vi "MegaAwesome_9_21_12a_JW.vi"() -> ()   [LabVIEW 2011]
uses:
  MegaAwesome_States.ctl
  <vilib>/Utility/inputDevices.llb/keyboardAcquire.vi
  <vilib>/Utility/file.llb/Read From Spreadsheet File (string).vi
  <vilib>/Utility/file.llb/Write To Spreadsheet File (string).vi
panel:
  out "ROI Descriptor out":T1 {"Contours"."Type" items=["No Selection", "Point", "Line", "Rectangle", "Oval", "Polygon", "Freehand Region", "Annulus", "Unused2", "Unused3", "Broken Line", "Freehand Line", "Rotated Rectangle"]}
  out "ROI Descriptor":T1 {"Contours"."Type" items=["No Selection", "Point", "Line", "Rectangle", "Oval", "Polygon", "Freehand Region", "Annulus", "Unused2", "Unused3", "Broken Line", "Freehand Line", "Rotated Rectangle"]}
  in  "Slider Min":dbl=5.0
  in  "Slider Max":dbl=5.0
  out "Opj X Axis":string
  out "X Axis Display Type":string
  in  "Index-Sat":dbl=5.0
  in  "Index-Lin":dbl=5.0
  in  "IndexLog-Lin":dbl=5.0
  in  "IndexLog-Sat":dbl=5.0 caption="Num Pts"
  out "Lin Id-Log Used":dbl[](array[numeric])
  out "Lin-Vg Array-Log Used":dbl[](array[numeric])
  in  "New: Comments":string
  out "Save Array":string[][](array[string])
  out "Folder Index":i32 caption="Length"
  out "Sat Id-Used":dbl[](array[numeric])
  out "Sat Vg Array-Used":dbl[](array[numeric])
  out "Vg Array-Log-Used":dbl[](array[numeric])
  out "Sat Id-Log-Used":dbl[](array[numeric])
  out "Lin Id-Used":dbl[](array[numeric])
  out "Lin-Vg Array-Used":dbl[](array[numeric])
  out "Lin Vd":dbl
  out "Recorded Prop":T2
  out "Current State":T3
  in  "Main Tab Control":T4(tab)
  in  "Image Analysis?":bool
  in  "Image Folder":path
  out "Image File":path=path "D:/UserData/Desktop/Jeremy/WFU/Research/Programs/VI mods/Image Not Found.png"
  in  "Transfer File":path
  out "Transfer Folder":path
  out "Fabrication Prop":T5
  in  "Transport ?":bool
  out "Distances":dbl[](array[numeric])
  in  "Zoom":i16(slide)=-3 scale=-5.0..5.0
  in  "Magnification":u16(ring) items=["5x", "10x", "20x", "50x", "80x"]
  in  "Undo Button":bool
  in  "Remove Button":bool
  in  "Transfer Plots":T6(tab)=enum."Saturation"
  in  "Lin-Trans Slider":dbl(slide) step=1.0 scale=-40.0..40.0 scale format="%#_1p"
  out "Sqrt-Lin":cluster{dbl[], dbl[]}[](graph)
  in  "Sat-Trans Slider":dbl(slide) step=1.0 scale=-40.0..40.0 scale format="%#_1p"
  out "Sqrt-Sat":cluster{dbl[], dbl[]}[](graph)
  out "Raw- Lin":cluster{dbl[], dbl[]}[](graph)
  out "Raw- Sat":cluster{dbl[], dbl[]}[](graph)
  in  "Log Plots":enum32{"Linear", "Saturation", "Transport"}(tab)=enum."Saturation"
  in  "Lin-Log Slider":dbl(slide) step=1.0 scale=-40.0..40.0 scale format="%#_1p"
  out "Log-Lin":cluster{dbl[], dbl[]}[](graph)
  in  "Sat-Log Slider":dbl(slide) step=1.0 scale=-40.0..40.0 scale format="%#_1p"
  out "Sat-Log":cluster{dbl[], dbl[]}[](graph)
  out "Transport":cluster{dbl[], dbl[]}[](graph)
  in  "Manual Controls":T7
  in  "File Controls":T8
  out "Date Recorded":string="Date Recorded" caption="Measured"
  out "Data Name:":string
  out "Image Name":string
  out "Index":string
  out "Date Created":string caption="Fabricated"
  in  "Comments:":string
  out "Rec: Length":dbl caption="Length" format="%#_3g"
  out "Rec: Width":dbl caption="Width" format="%#_4g"
  out "Rec: Dielectric (d)":dbl caption="Dielectric (d)" format="%#_3g"
  in  "New: Dielectric":dbl
  in  "New: Length":dbl
  in  "New: Width":dbl
  out "Rec: Temp":dbl caption="Sample Temp" format="%.1f"
  in  "New: Temp":dbl format="%.1f"
  out "Image Out":T9(plugin-control)
  in  "Num Pts":dbl=5.0
  in  "Num Pts Log":dbl=5.0 caption="Num Pts"
  out "Recorded Values Cluster":T10
  out "Calculated Values Cluster":T10 caption="Recorded Values Cluster"
  out "Re-Calculated Values Cluster":T10 caption="Recorded Values Cluster"
  in  "Independant Variable:":string(combo)="Length (um):"
  out "Image Preview":T9(plugin-control)
  out "Total Width":dbl
  in  "No Image File":path=path "\\\\acad1\\physics/Jurchescu-group/JW-PD/Mega Awesome/Image Not Found.png"
  in  "Room Temp":dbl=294.0
  in  "Origin Project File":path=path "\\\\acad1\\physics/Jurchescu-group/JW-PD/Group Library/Origin Project Files/DeviceData_8_10_12a_JW.opj"
  in  "Transport Style Controls":T11={"Transport Line Size"=1, "Transport Line Color"=16772608} {"Transport Line Size" items=["Extra Small", "Small", "Medium", "Large", "Extra Large"]}
  # "Image Location"
  # "Recorded"
  # "Calculated"
  # "Re-Calculated"
  # "Manual"
  # "Used points display at y=0\nValues are wrong w/ slider"
  # "Slider\nDoesn't\nWork"
  # "Slider\nDoesn't\nWork"
  # "No new points displayed"
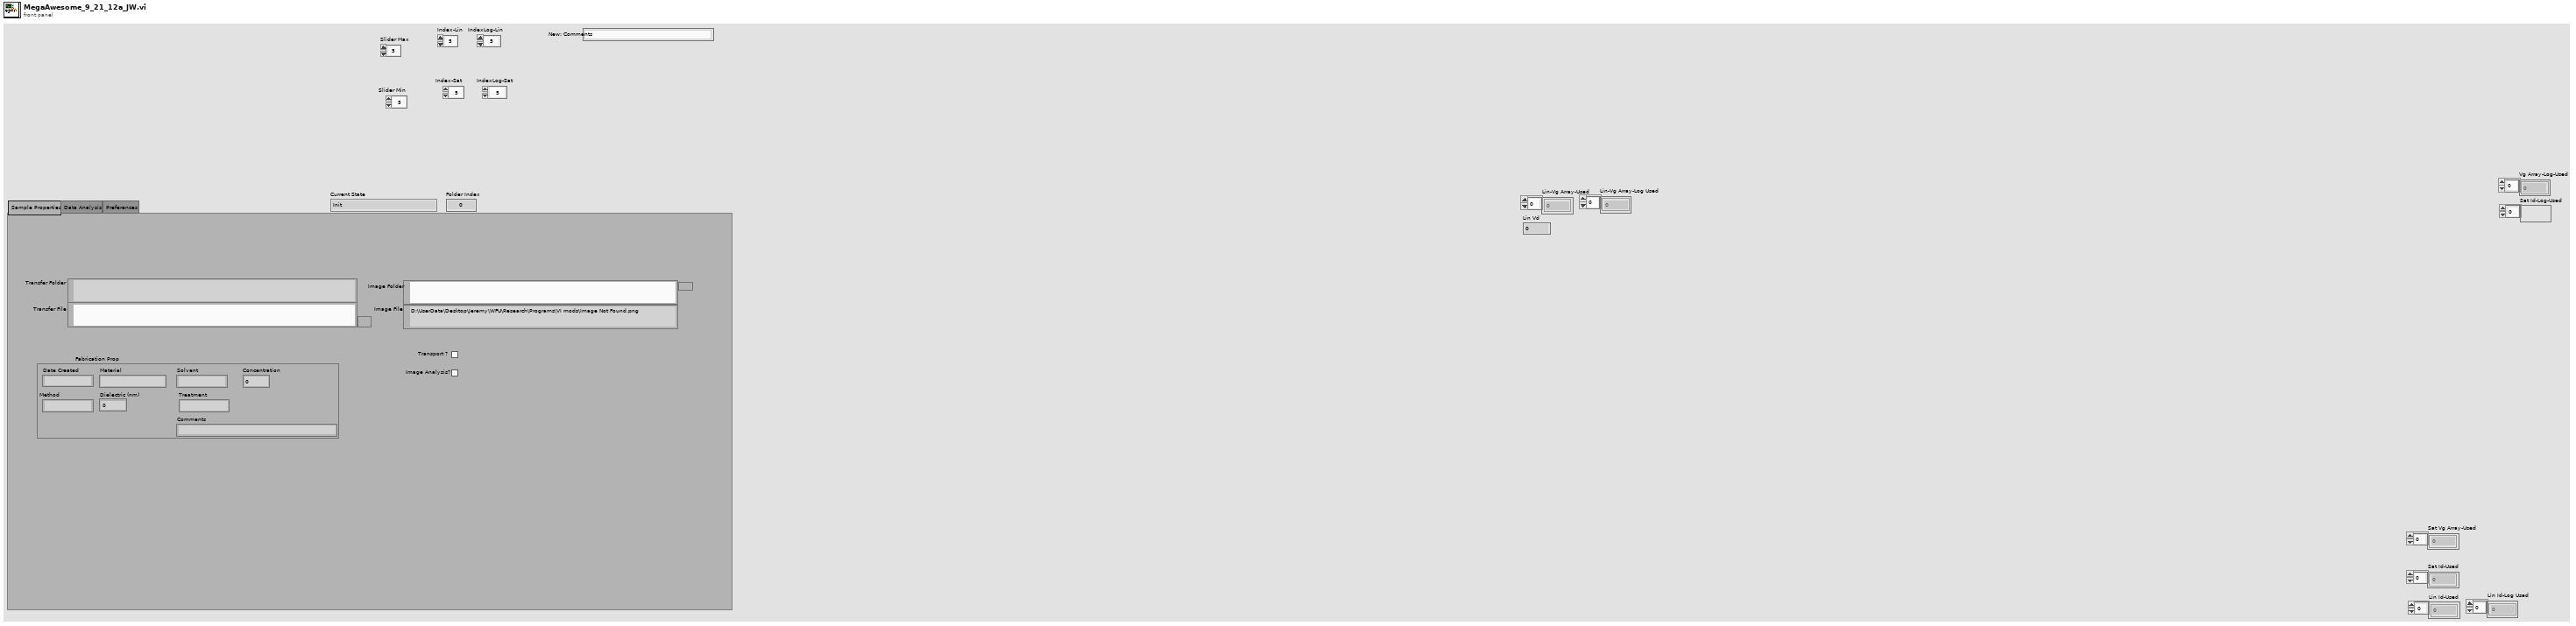
[diagram p1: front panel]
types:
  T1 = typedef "ROI Descriptor" = cluster{"Global Rectangle":i32[], "Contours":cluster{"ID":enum32{"External", "Internal"}, "Type":u32, "Coordinates":i32[]}[]}
  T2 = cluster{"Date Recorded":string, "Index":string, "Length":dbl, "Width":dbl, "Sample Temp":dbl}
  T3 = typedef "MegaAwesome_States.ctl" = enum16{"Init", "File Missing", "No Event", "Read Data", "Calculated Values", "Re-Calculated Values", "Next File", "Previous File", "Discard File", "Save", "Save Lines", "Export", "Exit"}
  T4 = enum32{"Sample Properties", "Data Analysis", "Preferences"}
  T5 = cluster{"Date Created":string, "Material":string, "Solvent":string, "Concentration":dbl, "Method":string, "Dielectric (nm)":dbl, "Treatment":string, "Comments":string}
  T6 = enum32{"Linear", "Saturation", "Raw-Linear", "Raw-Saturation"}
  T7 = cluster{"Manual-Temp":bool, "Manual-Width":bool, "Manuel-Length":bool, "Manuel-Dielectric":bool, "Manual Comments":bool}
  T8 = cluster{"Previous File":bool, "Discard ":bool, "Save Lines":bool, "Close":bool, "Next File ":bool, "Save":bool, "Save Next":bool, "Export":bool}
  T9 = typedef "IMAQ Image.ctl" = refnum<image>
  T10 = cluster{"Mobility-Sat":dbl, "Moblitity-Lin":dbl, "On/Off":dbl, "Off Current":dbl, "Vt-Sat":dbl, "STS":dbl, "Trap Density-VT":dbl, "Trap Density-STS":dbl}
  T11 = cluster{"Transport Line Size":u16, "Transport Line Color":u32}
  T12 = typedef "LVBoundsTypeDef.ctl" = cluster{"Width":u32, "Height":u32}
  T13 = cluster{"Global Rectangle":i32[], "Contours":cluster{"Contour Type":u32, "ROI Type":u32, "Points":i32[]}[]}
  T14 = cluster{"Contour Type":u32, "ROI Type":u32, "Points":i32[]}[]
  T15 = cluster{i32[], cluster{"Contour Type":u32, "ROI Type":u32, "Points":i32[]}[]}
  T16 = enum16{"0", "1", "2", "3", "4", "5", "6", "7", "8", "9", "A", "B", "C", "D", "E", "F", "G", "H", "I", "J", "K", "L", "M", "N", "O", "P", "Q", "R", "S", "T", "U", "V", "W", "X", "Y", "Z", "F1", "F2", "F3", "F4", "F5", "F6", "F7", "F8", "F9", "F10", "F11", "F12", "F13", "F14", "F15", "ADD", "BACK", "BACKSLASH", "CAPITAL", "COMMA", "DECIMAL", "DELETE", "DIVIDE", "DOWN", "END", "EQUALS", "ESCAPE", "GRAVE (`)", "HOME", "INSERT", "LBRACKET", "LCONTROL", "LEFT", "L ALT", "LSHIFT", "LWIN", "MINUS", "MULTIPLY", "NEXT", "NUMLOCK", "NUMPAD_0", "NUMPAD_1", "NUMPAD_2", "NUMPAD_3", "NUMPAD_4", "NUMPAD_5", "NUMPAD_6", "NUMPAD_7", "NUMPAD_8", "NUMPAD_9", "PAUSE", "PERIOD", "PRIOR (PG UP)", "RBRACKET", "RCONTROL", "RETURN", "RIGHT", "R ALT", "RSHIFT", "RWIN", "SCROLL", "SEMICOLON", "SLASH", "SPACE", "SUBTRACT", "TAB", "UP", "ENTER (num pad)", "' (quote)"}[]
  T17 = enum16{"0", "1", "2", "3", "4", "5", "6", "7", "8", "9", "A", "B", "C", "D", "E", "F", "G", "H", "I", "J", "K", "L", "M", "N", "O", "P", "Q", "R", "S", "T", "U", "V", "W", "X", "Y", "Z", "F1", "F2", "F3", "F4", "F5", "F6", "F7", "F8", "F9", "F10", "F11", "F12", "F13", "F14", "F15", "ADD", "BACK", "BACKSLASH", "CAPITAL", "COMMA", "DECIMAL", "DELETE", "DIVIDE", "DOWN", "END", "EQUALS", "ESCAPE", "GRAVE (`)", "HOME", "INSERT", "LBRACKET", "LCONTROL", "LEFT", "L ALT", "LSHIFT", "LWIN", "MINUS", "MULTIPLY", "NEXT", "NUMLOCK", "NUMPAD_0", "NUMPAD_1", "NUMPAD_2", "NUMPAD_3", "NUMPAD_4", "NUMPAD_5", "NUMPAD_6", "NUMPAD_7", "NUMPAD_8", "NUMPAD_9", "PAUSE", "PERIOD", "PRIOR (PG UP)", "RBRACKET", "RCONTROL", "RETURN", "RIGHT", "R ALT", "RSHIFT", "RWIN", "SCROLL", "SEMICOLON", "SLASH", "SPACE", "SUBTRACT", "TAB", "UP", "ENTER (num pad)", "' (quote)"}
  T18 = cluster{string, sgl, bool, bool, bool, bool, bool, bool, i32}
  T19 = cluster{i32, cluster{string, sgl, bool, bool, bool, bool, bool, bool, i32}, i32, i32}
  T20 = cluster{"Contour Type":u32, "ROI Type":u32, "Points":i32[]}
  T21 = cluster{"Points[0]":i32, "Points[1]":i32, "Points[2]":i32, "Points[3]":i32, "Points[4]":i32, "Points[5]":i32, "Points[6]":i32, "Points[7]":i32, "Points[8]":i32}
  T22 = cluster{"[0]":cluster{dbl[], dbl[]}, "[1]":cluster{dbl[], dbl[]}, "[2]":cluster{dbl[], dbl[]}, "[3]":cluster{dbl[], dbl[]}, "[4]":cluster{dbl[], dbl[]}, "[5]":cluster{dbl[], dbl[]}, "[6]":cluster{dbl[], dbl[]}, "[7]":cluster{dbl[], dbl[]}, "[8]":cluster{dbl[], dbl[]}}
  T23 = cluster{"Sat Vg Used":dbl[], "Sat Sqrt(Id) Used ":dbl[], "Lin Vg Used":dbl[], "Lin Sqrt(Id) Used":dbl[], "Index-Lin":dbl, "Index-Sat":dbl}
  T24 = cluster{"Raw Sat":cluster{dbl[], dbl[]}[], "Sqrt Sat":cluster{dbl[], dbl[]}[], "Log Sat":cluster{dbl[], dbl[]}[], "Raw Lin":cluster{dbl[], dbl[]}[], "Sqrt Lin":cluster{dbl[], dbl[]}[], "Log Lin":cluster{dbl[], dbl[]}[]}
  T25 = cluster{"Mobility-Sat":dbl, "Vt-Sat":dbl, "Mobility-Lin":dbl, "Vt-Lin":dbl, "Off I-Sat":dbl, "On/Off I-Sat":dbl}
  T26 = cluster{"Sat Vg Used":dbl[], "Sat Log(Id) Used":dbl[], "Lin Vg Used":dbl[], "Lin Log(Id) Used":dbl[], "STS Index-Sat":dbl, "STS Index-Lin":dbl}
  T27 = cluster{"Independant  Variable Indicator":string, "Parameter String Indicator":string}
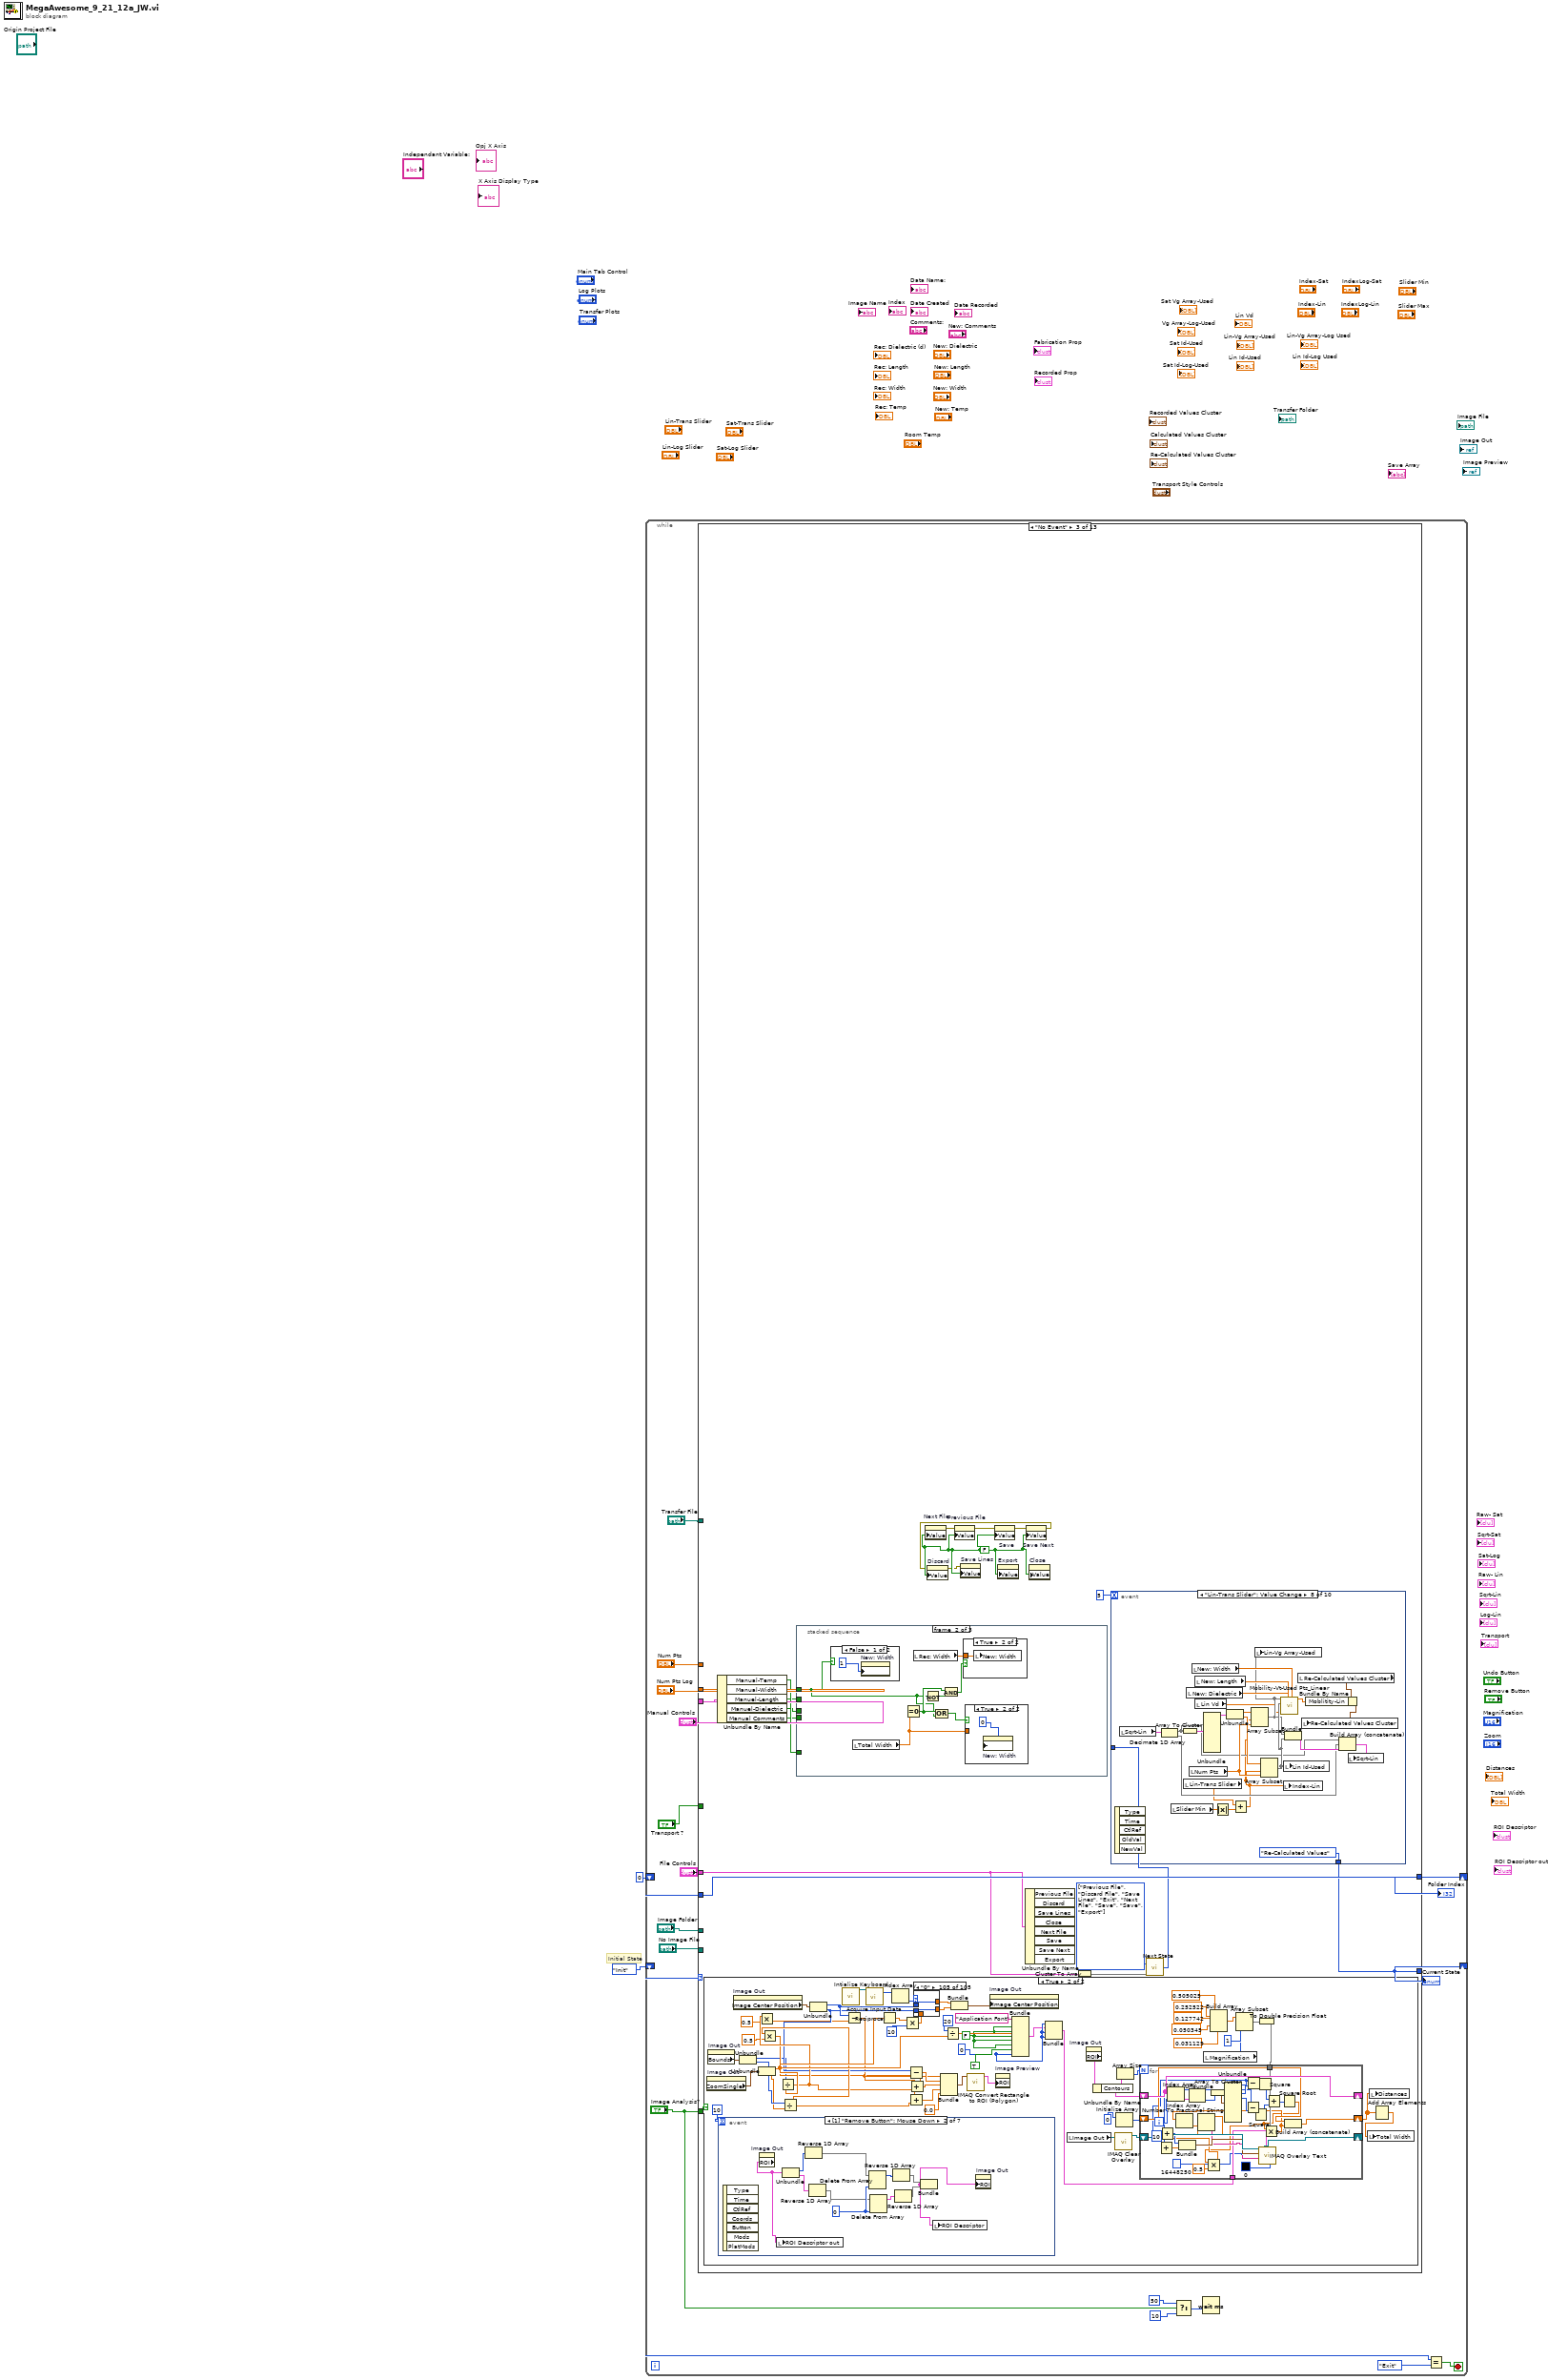
[diagram p0: block diagram]
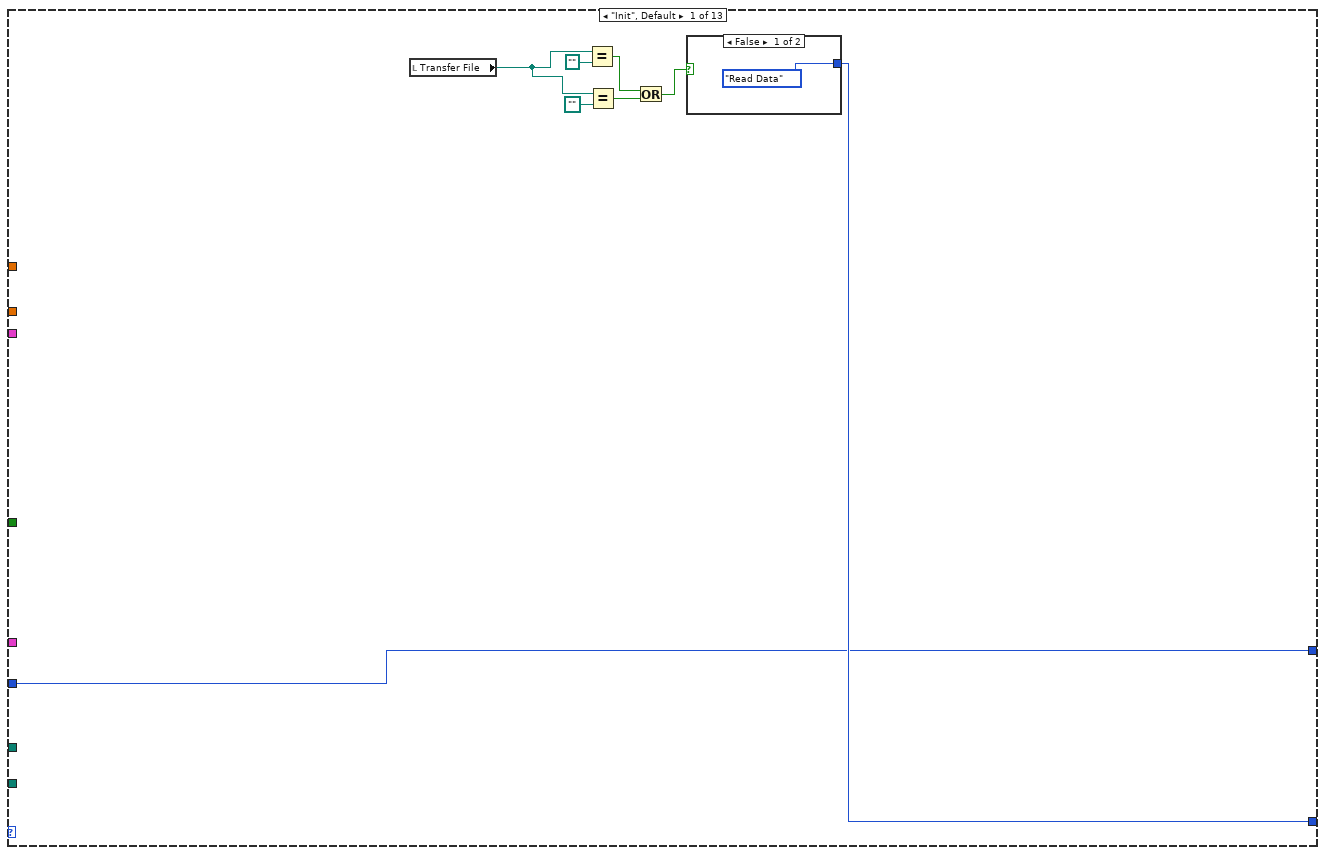
[diagram p2: hidden frame]
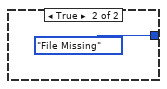
[diagram p3: hidden frame]
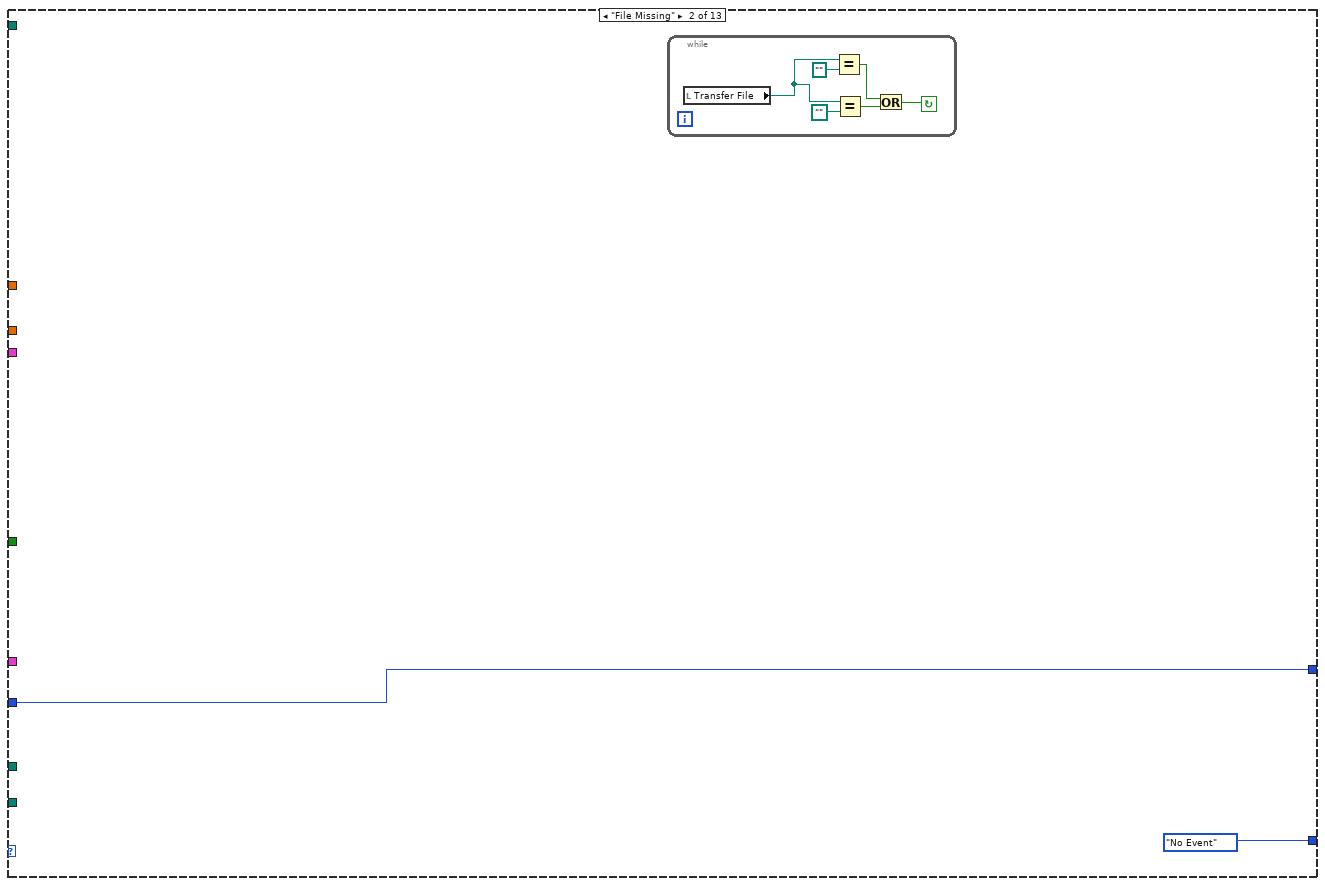
[diagram p4: hidden frame]
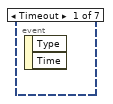
[diagram p6: hidden frame]
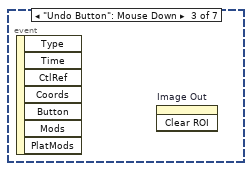
[diagram p7: hidden frame]
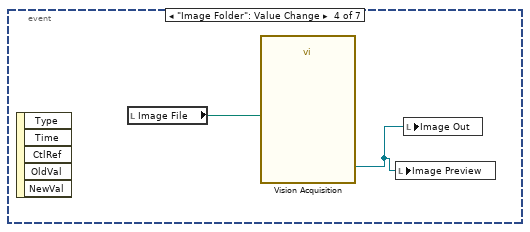
[diagram p8: hidden frame]
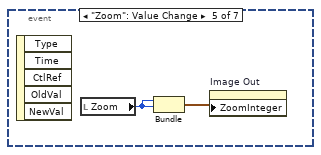
[diagram p9: hidden frame]
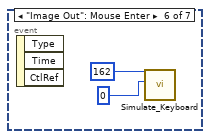
[diagram p10: hidden frame]
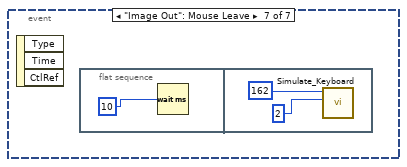
[diagram p11: hidden frame]
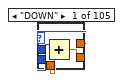
[diagram p12: hidden frame]
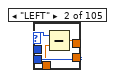
[diagram p13: hidden frame]
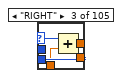
[diagram p14: hidden frame]
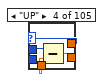
[diagram p15: hidden frame]
diagram:
  # "Initial State"
  n1 = while {
    shift-right: [w17] -> _
    shift-left: MegaAwesome_States."Init" -> [w19]
    shift-right: [w10] -> _
    shift-left: 0 -> [w11]
    stop <- w20 stop-if-true
    n2 = case shown="\"No Event\"" w19 {
      tunnel: [w22 MegaAwesome_States."No Event" w48 MegaAwesome_States."Calculated Values" MegaAwesome_States."Re-Calculated Values" MegaAwesome_States."No Event" MegaAwesome_States."Read Data" MegaAwesome_States."Read Data" MegaAwesome_States."No Event" w677 MegaAwesome_States."No Event" MegaAwesome_States."No Event" MegaAwesome_States."Exit"] -> w17
      tunnel: "Transfer File" -> [_ _ _ w522 w557 _ w646 w658 _ w682 _ _ _]
      tunnel: "Num Pts" -> [_ _ _ _ w581 _ _ _ _ _ _ _ _]
      tunnel: "Num Pts Log" -> [_ _ _ _ w580 _ _ _ _ _ _ _ _]
      tunnel: "Image Folder" -> [_ _ _ _ w577 _ _ _ _ _ _ _ _]
      tunnel: "No Image File" -> [_ _ _ _ w576 _ _ _ _ _ _ _ _]
      tunnel: [w21 w31 w56 w516 w575 w606 w631 w656 w674 w683 w1198 w1201 w1202] -> w10
      tunnel: w11 -> [w21 w31 w56 _ w575 w606 w632 w657 w674 w683 w1198 w1201 w1202]
      tunnel: "Manual Controls" -> [_ _ w50 _ _ _ _ _ _ w681 _ _ _]
      tunnel: "File Controls" -> [_ _ w46 _ _ _ _ _ _ w676 _ _ _]
      tunnel: "Transport ?" -> [_ _ _ _ w543 _ _ _ _ _ _ _ _]
      tunnel: "Image Analysis?" -> [_ _ w39 _ _ _ _ _ _ _ _ _ _]
      frame "Init", Default {
        n3 = local read "Transfer File"() -> (w23:path)
        n4 = Equal?(x=w23, y=path "") -> (x = y?=w26:bool)
        n5 = Equal?(x=w23, y=path "") -> (x = y?=w25:bool)
        n6 = Or(x=w26, y=w25) -> (x .or. y?=w28:bool)
        n7 = case shown="False" w28 {
          tunnel: [MegaAwesome_States."Read Data" MegaAwesome_States."File Missing"] -> w22
          frame False {
          }
          frame True {
          }
        }
      }
      frame "File Missing" {
        n8 = while {
          stop <- w33 continue-if-true
          n9 = local read "Transfer File"() -> (w34:path)
          n10 = Equal?(x=w34, y=path "") -> (x = y?=w36:bool)
          n11 = Equal?(x=w34, y=path "") -> (x = y?=w37:bool)
          n12 = Or(x=w36, y=w37) -> (x .or. y?=w33:bool)
        }
      }
      frame "No Event" {
        w45 = FALSE
        w58 = T3[] [enum."Previous File", enum."Discard File", enum."Save Lines", enum."Exit", enum."Next File", enum."Save", enum."Save", enum."Export"] items=["Init", "File Missing", "No Event", "Read Data", "Calculated Values", "Re-Calculated Values", "Next File", "Previous File", "Discard File", "Save", "Save Lines", "Export", "Exit"]
        n13 = case shown="True" w39 {
          frame False {
          }
          frame True {
            w108 = FALSE
            w110 = 0
            n14 = property on="Image Out" class="ImageControl"() -> ("ZoomSingle"=w93:cluster{"X":sgl, "Y":sgl})  [unwired: 2 in, 2 out]
            n15 = property on="Image Out" class="ImageControl"() -> ("Bounds"=w92:T12)  [unwired: 2 in, 2 out]
            n16 = event shown="[1] \"Remove Button\": Mouse Down" {
              selector: _ -> [_ _ _ _ _ _ _]
              dyn-events: _ -> [_ _ _ _ _ _ _]
              timeout: 10 -> [_ _ _ _ _ _ _]
              event Timeout {
                n17 = event-data() -> ()  [unwired: 1 in, 2 out]
              }
              event "Remove Button": Mouse Down {
                w128 = 0
                n18 = event-data() -> ()  [unwired: 1 in, 7 out]
                n19 = property on="Image Out" class="ImageControl"() -> ("ROI"=w118:T13)  [unwired: 2 in, 2 out]
                n20 = local write "ROI Descriptor out"(w118) -> ()
                n21 = Unbundle(w118) -> ("Global Rectangle"=w127:i32[], "Contours"=w125:T14)
                n22 = Reverse 1D Array(array=w127) -> (reversed array=w126:i32[])
                n23 = Reverse 1D Array(array=w125) -> (reversed array=w124:T14)
                n24 = Delete From Array(array=w126, index=w128) -> (array with subset deleted=w123:i32[])  [unwired: 1 in, 1 out]
                n25 = Delete From Array(array=w124, index=w128) -> (array with subset deleted=w122:T14)  [unwired: 1 in, 1 out]
                n26 = Reverse 1D Array(array=w123) -> (reversed array=w121:i32[])
                n27 = Reverse 1D Array(array=w122) -> (reversed array=w120:T14)
                n28 = Bundle(w121, w120) -> (w119:T15)  [unwired: 1 in]
                n29 = local write "ROI Descriptor"(w119) -> ()
                n30 = property on="Image Out" class="ImageControl"("ROI"=w119) -> ()  [unwired: 2 in, 2 out]
              }
              event "Undo Button": Mouse Down {
                n31 = event-data() -> ()  [unwired: 1 in, 7 out]
                n32 = invoke on="Image Out" class="ImageControl" method="Clear ROI"() -> ()  [unwired: 3 in, 3 out]
              }
              event "Image Folder": Value Change {
                n33 = event-data() -> ()  [unwired: 1 in, 5 out]
                n34 = local read "Image File"() -> (w130:path)
                n35 = call "Vision Acquisition"("Image Path"=w130) -> ("Image Out"=w129:T9)  [unwired: 25 in, 1 out]
                n36 = local write "Image Preview"(w129) -> ()
                n37 = local write "Image Out"(w129) -> ()
              }
              event "Zoom": Value Change {
                n38 = event-data() -> ()  [unwired: 1 in, 5 out]
                n39 = local read "Zoom"() -> (w131:i16)
                n40 = Bundle("Zoom"=w131, "Zoom"=w131) -> (w132:cluster{"Zoom":i16, "Zoom":i16})  [unwired: 1 in]
                n41 = property on="Image Out" class="ImageControl"("ZoomInteger"=w132) -> ()  [unwired: 2 in, 2 out]
              }
              event "Image Out": Mouse Enter {
                n42 = event-data() -> ()  [unwired: 1 in, 3 out]
                n43 = call "Simulate_Keyboard.vi"("Action"=0, "Virtual Key"=162) -> ()  [unwired: 7 in, 1 out]
              }
              event "Image Out": Mouse Leave {
                n44 = event-data() -> ()  [unwired: 1 in, 3 out]
                n45 = flat-sequence {
                  frame #0 {
                    n46 = Wait (ms)(milliseconds to wait=10) -> ()  [unwired: 1 out]
                  }
                  frame #1 {
                    n47 = call "Simulate_Keyboard.vi"("Action"=2, "Virtual Key"=162) -> ()  [unwired: 7 in, 1 out]
                  }
                }
              }
            }
            n48 = property on="Image Out" class="ImageControl"() -> ("Image Center Position"=w86:cluster{"X":u32, "Y":u32})  [unwired: 2 in, 2 out]
            n49 = Unbundle(w92) -> ("Width"=w95:u32, "Height"=w96:u32)
            n50 = Unbundle(w93) -> ("X"=w115:sgl, "Y"=w94:sgl)
            n51 = Divide(x=w95, y=w115) -> (x/y=w105:sgl)
            n52 = Multiply(x=w105, y=0.5) -> (x*y=w99:dbl)
            n53 = Divide(x=w96, y=w94) -> (x/y=w106:sgl)
            n54 = Multiply(x=w106, y=0.5) -> (x*y=w100:dbl)
            n55 = Unbundle(w86) -> ("X"=w104:u32, "Y"=w103:u32)
            n56 = call <vilib>:"Intialize Keyboard.vi"() -> ("device ID"=w83:refnum<k1>)  [unwired: 10 in, 1 out]
            n57 = Subtract(x=w104, y=w99) -> (x-y=w101:dbl)
            n58 = call-poly <vilib>:"Acquire Input Data.vi"("device ID"=w83) -> ("keys pressed"=w84:T16)  [unwired: 16 in, 2 out]
            n59 = Reciprocal(x=w115) -> (1/x=w116:sgl)
            n60 = Index Array(array=w84) -> (element=w80:T17)  [unwired: 1 in]
            n61 = Multiply(x=w116, y=10) -> (x*y=w114:sgl)
            n62 = Subtract(x=w103, y=w100) -> (x-y=w102:dbl)
            n63 = Add(x=w102, y=w106) -> (x+y=w88:dbl)
            n64 = Add(x=w101, y=w105) -> (x+y=w87:dbl)
            n65 = case shown="\"0\"" w80 {
              tunnel: w104 -> [w171 w177 w181 w183 w187 w189 w191 w193 w195 w197 w199 w201 w203 w205 w207 w209 w211 w213 w215 w217 w219 w221 w223 w225 w227 w229 w231 w233 w235 w237 w239 w241 w243 w245 w247 w249 w251 w253 w255 w257 w259 w261 w263 w265 w267 w269 w271 w273 w275 w277 w279 w281 w283 w285 w287 w289 w291 w293 w295 w297 w299 w301 w303 w305 w307 w309 w311 w313 w315 w317 w319 w321 w323 w325 w327 w329 w331 w333 w335 w337 w339 w341 w343 w345 w347 w349 w351 w353 w355 w357 w359 w361 w363 w365 w367 w369 w371 w373 w375 w377 w379 w381 w383 w385 w387]
              tunnel: [w171 w176 w180 w183 w187 w189 w191 w193 w195 w197 w199 w201 w203 w205 w207 w209 w211 w213 w215 w217 w219 w221 w223 w225 w227 w229 w231 w233 w235 w237 w239 w241 w243 w245 w247 w249 w251 w253 w255 w257 w259 w261 w263 w265 w267 w269 w271 w273 w275 w277 w279 w281 w283 w285 w287 w289 w291 w293 w295 w297 w299 w301 w303 w305 w307 w309 w311 w313 w315 w317 w319 w321 w323 w325 w327 w329 w331 w333 w335 w337 w339 w341 w343 w345 w347 w349 w351 w353 w355 w357 w359 w361 w363 w365 w367 w369 w371 w373 w375 w377 w379 w381 w383 w385 w387] -> w81
              tunnel: w103 -> [w173 w175 w179 w185 w186 w188 w190 w192 w194 w196 w198 w200 w202 w204 w206 w208 w210 w212 w214 w216 w218 w220 w222 w224 w226 w228 w230 w232 w234 w236 w238 w240 w242 w244 w246 w248 w250 w252 w254 w256 w258 w260 w262 w264 w266 w268 w270 w272 w274 w276 w278 w280 w282 w284 w286 w288 w290 w292 w294 w296 w298 w300 w302 w304 w306 w308 w310 w312 w314 w316 w318 w320 w322 w324 w326 w328 w330 w332 w334 w336 w338 w340 w342 w344 w346 w348 w350 w352 w354 w356 w358 w360 w362 w364 w366 w368 w370 w372 w374 w376 w378 w380 w382 w384 w386]
              tunnel: [w172 w175 w179 w184 w186 w188 w190 w192 w194 w196 w198 w200 w202 w204 w206 w208 w210 w212 w214 w216 w218 w220 w222 w224 w226 w228 w230 w232 w234 w236 w238 w240 w242 w244 w246 w248 w250 w252 w254 w256 w258 w260 w262 w264 w266 w268 w270 w272 w274 w276 w278 w280 w282 w284 w286 w288 w290 w292 w294 w296 w298 w300 w302 w304 w306 w308 w310 w312 w314 w316 w318 w320 w322 w324 w326 w328 w330 w332 w334 w336 w338 w340 w342 w344 w346 w348 w350 w352 w354 w356 w358 w360 w362 w364 w366 w368 w370 w372 w374 w376 w378 w380 w382 w384 w386] -> w82
              tunnel: w114 -> [w170 w174 w178 w182 _ _ _ _ _ _ _ _ _ _ _ _ _ _ _ _ _ _ _ _ _ _ _ _ _ _ _ _ _ _ _ _ _ _ _ _ _ _ _ _ _ _ _ _ _ _ _ _ _ _ _ _ _ _ _ _ _ _ _ _ _ _ _ _ _ _ _ _ _ _ _ _ _ _ _ _ _ _ _ _ _ _ _ _ _ _ _ _ _ _ _ _ _ _ _ _ _ _ _ _ _]
              frame "DOWN" {
                n66 = Add(x=w173, y=w170) -> (x+y=w172:sgl)
              }
              frame "LEFT" {
                n67 = Subtract(x=w177, y=w174) -> (x-y=w176:sgl)
              }
              frame "RIGHT" {
                n68 = Add(x=w181, y=w178) -> (x+y=w180:sgl)
              }
              frame "UP" {
                n69 = Subtract(x=w185, y=w182) -> (x-y=w184:sgl)
              }
              frame "ENTER (num pad)" {
              }
              frame "' (quote)" {
              }
              frame "END" {
              }
              frame "EQUALS" {
              }
              frame "ESCAPE" {
              }
              frame "GRAVE (`)" {
              }
              frame "HOME" {
              }
              frame "INSERT" {
              }
              frame "LBRACKET" {
              }
              frame "LCONTROL" {
              }
              frame "L ALT" {
              }
              frame "LSHIFT" {
              }
              frame "LWIN" {
              }
              frame "MINUS" {
              }
              frame "MULTIPLY" {
              }
              frame "NEXT" {
              }
              frame "NUMLOCK" {
              }
              frame "NUMPAD_0" {
              }
              frame "NUMPAD_1" {
              }
              frame "NUMPAD_2" {
              }
              frame "NUMPAD_3" {
              }
              frame "NUMPAD_4" {
              }
              frame "NUMPAD_5" {
              }
              frame "NUMPAD_6" {
              }
              frame "NUMPAD_7" {
              }
              frame "NUMPAD_8" {
              }
              frame "NUMPAD_9" {
              }
              frame "PAUSE" {
              }
              frame "PERIOD" {
              }
              frame "PRIOR (PG UP)" {
              }
              frame "RBRACKET" {
              }
              frame "RCONTROL" {
              }
              frame "RETURN" {
              }
              frame "R ALT" {
              }
              frame "RSHIFT" {
              }
              frame "RWIN" {
              }
              frame "SCROLL" {
              }
              frame "SEMICOLON" {
              }
              frame "SLASH" {
              }
              frame "SPACE" {
              }
              frame "SUBTRACT" {
              }
              frame "TAB" {
              }
              frame "DIVIDE" {
              }
              frame "DELETE" {
              }
              frame "DECIMAL" {
              }
              frame "COMMA" {
              }
              frame "CAPITAL" {
              }
              frame "BACKSLASH" {
              }
              frame "BACK" {
              }
              frame "ADD" {
              }
              frame "F15" {
              }
              frame "F14" {
              }
              frame "F13" {
              }
              frame "F12" {
              }
              frame "F11" {
              }
              frame "F10" {
              }
              frame "F9" {
              }
              frame "F8" {
              }
              frame "F7" {
              }
              frame "F6" {
              }
              frame "F5" {
              }
              frame "F4" {
              }
              frame "F3" {
              }
              frame "F2" {
              }
              frame "F1" {
              }
              frame "Z" {
              }
              frame "Y" {
              }
              frame "X" {
              }
              frame "W" {
              }
              frame "V" {
              }
              frame "U" {
              }
              frame "T" {
              }
              frame "S" {
              }
              frame "R" {
              }
              frame "Q" {
              }
              frame "P" {
              }
              frame "O" {
              }
              frame "N" {
              }
              frame "M" {
              }
              frame "L" {
              }
              frame "K" {
              }
              frame "J" {
              }
              frame "I" {
              }
              frame "H" {
              }
              frame "G" {
              }
              frame "F" {
              }
              frame "E" {
              }
              frame "D" {
              }
              frame "C" {
              }
              frame "B" {
              }
              frame "A" {
              }
              frame "9" {
              }
              frame "8" {
              }
              frame "7" {
              }
              frame "6" {
              }
              frame "5" {
              }
              frame "4" {
              }
              frame "3" {
              }
              frame "2" {
              }
              frame "1" {
              }
              frame "0" {
              }
            }
            n70 = Bundle(w101, w102, w87, w88, 0.0) -> (w89:cluster{dbl, dbl, dbl, dbl, dbl})  [unwired: 1 in]
            n71 = Divide(x=20, y=w115) -> (x/y=w112:sgl)
            n72 = Bundle("X"=w81, "Y"=w82) -> (w85:cluster{"X":sgl, "Y":sgl})  [unwired: 1 in]
            n73 = call "IMAQ Convert Rectangle to ROI (Polygon)"("Rectangle"=w89) -> ("ROI Descriptor"=w91:T1)  [unwired: 7 in, 2 out]
            n74 = property on="Image Out" class="ImageControl"("Image Center Position"=w85) -> ()  [unwired: 2 in, 2 out]
            n75 = property on="Image Preview" class="ImageControl"("ROI"=w91) -> ()  [unwired: 2 in, 2 out]
            n76 = Bundle("Application Font", w112, w108, w108, w108, w108, w108, TRUE, w110) -> (w107:T18)  [unwired: 1 in]
            n77 = Bundle(w110, w107, w110, w110) -> (w61:T19)  [unwired: 1 in]
            n78 = local read "Image Out"() -> (w60:T9)
            n79 = property on="Image Out" class="ImageControl"() -> ("ROI"=w64:T13)  [unwired: 2 in, 2 out]
            n80 = Unbundle By Name(w64) -> ("Contours"=w65:T14)
            n81 = call "IMAQ Clear Overlay"("Image"=w60) -> ("Image Out"=w79:T9)  [unwired: 9 in, 1 out]
            n82 = Initialize Array(0) -> (w67:i32[])  [unwired: 1 in]
            n83 = Array Size(array=w65) -> (size(s)=w66:i32)
            n84 = local read "Magnification"() -> (w75:u16)
            n85 = Build Array(0.505025, 0.252522, 0.127742, 0.050345, 0.031129) -> (w74:dbl[])
            n86 = Array Subset(array=w74, index=w75, length=1) -> (w77:dbl[])
            n87 = To Double Precision Float(number=w77) -> (double precision float=w78:dbl[])
            n88 = for {
              N: w66 -> [_]
              shift-right: [w160] -> _
              shift-left: w65 -> [w160]
              shift-right: [w158] -> w62
              shift-left: w67 -> [w157]
              tunnel: w78 -> [w156]
              shift-right: [w153] -> _
              shift-left: w79 -> [w155]
              tunnel: w61 -> [w148]
              i -> [w152]
              n89 = Index Array(array=w160, index=w152) -> (element=w169:T20)
              n90 = Unbundle(w169) -> ("Points"=w168:i32[])  [unwired: 2 out]
              n91 = Array To Cluster(array=w168) -> (cluster=w167:T21)
              n92 = Unbundle(w167) -> ("Points[0]"=w147:i32, "Points[1]"=w144:i32, "Points[2]"=w159:i32, "Points[3]"=w165:i32)  [unwired: 5 out]
              n93 = Add(x=w147, y=10) -> (x+y=w145:i32)
              n94 = Subtract(x=w144, y=w165) -> (x-y=w164:i32)
              n95 = Subtract(x=w147, y=w159) -> (x-y=w166:i32)
              n96 = Square(x=w164) -> (x^2=w162:i32)
              n97 = Square(x=w166) -> (x^2=w163:i32)
              n98 = Add(x=w163, y=w162) -> (x+y=w161:i32)
              n99 = Square Root(x=w161) -> (sqrt(x)=w138:dbl)
              n100 = Multiply(x=w138, y=0.5) -> (x*y=w141:dbl)
              n101 = Add(x=w141, y=w144) -> (x+y=w143:dbl)
              n102 = Bundle(w145, w143) -> (w154:cluster{i32, dbl})  [unwired: 1 in]
              n103 = Multiply(x=w138, y=w156) -> (x*y=w151:dbl[])
              n104 = Index Array(array=w151) -> (element=w150:dbl)  [unwired: 1 in]
              n105 = Number To Fractional String(number=w150) -> (F-format string=w149:string)  [unwired: 3 in]
              n106 = call "IMAQ Overlay Text"("BG Color (Transparent)"=u32 0, "Text Color (black)"=u32 16448250, "Font, Size & Style"=w148, "String"=w149, "Origin"=w154, "Image"=w155) -> ("Image Out"=w153:T9)  [unwired: 4 in, 1 out]
              n107 = Build Array (concatenate)(w157, w151) -> (w158:dbl[])
            }
            n108 = local write "Distances"(w62) -> ()
            n109 = Add Array Elements(numeric array=w62) -> (sum=w63:dbl)
            n110 = local write "Total Width"(w63) -> ()
          }
        }
        n111 = Unbundle By Name(w50) -> ("Manual-Temp"=w55:bool, "Manual-Width"=w54:bool, "Manuel-Length"=w53:bool, "Manuel-Dielectric"=w52:bool, "Manual Comments"=w51:bool)
        n112 = stacked-sequence {
          tunnel: w55 -> [w480 _ _]
          tunnel: w54 -> [_ w490 _]
          tunnel: w53 -> [_ _ w505]
          tunnel: w52 -> [_ _ w502]
          tunnel: w51 -> [_ _ w501]
          frame #0 {
            n113 = local read "Rec: Temp"() -> (w479:dbl)
            n114 = case shown="False" w480 {
              tunnel: w479 -> [w485 _]
              tunnel: [w482 w489] -> _
              frame False {
                n115 = local read "Rec: Temp"() -> (w483:dbl)
                n116 = property on="New: Temp" class="DigNum (strict)"("DisabledEnum"=1) -> ()  [unwired: 2 in, 2 out]
                n117 = Equal To 0?(x=w483) -> (x = 0?=w484:bool)
                n118 = local write "New: Temp"(w485) -> ()
                n119 = case shown="True" w484 {
                  tunnel: [w486 w487] -> w482
                  tunnel: w483 -> [w486 _]
                  frame False {
                  }
                  frame True {
                    n120 = local read "Room Temp"() -> (w487:dbl)
                  }
                }
                n121 = local write "New: Temp"(w482) -> ()
              }
              frame True {
                n122 = property on="New: Temp" class="DigNum (strict)"("DisabledEnum"=0) -> ()  [unwired: 2 in, 2 out]
                n123 = local read "New: Temp"() -> (w489:dbl)
              }
            }
          }
          frame #1 {
            n124 = case shown="False" w490 {
              frame False {
                n125 = property on="New: Width" class="DigNum (strict)"("DisabledEnum"=1) -> ()  [unwired: 2 in, 2 out]
              }
              frame True {
                (unwired) 0
              }
            }
            n126 = local read "Total Width"() -> (w496:dbl)
            n127 = Equal To 0?(x=w496) -> (x = 0?=w493:bool)
            n128 = local read "Rec: Width"() -> (w494:dbl)
            n129 = Not(x=w490) -> (.not. x?=w492:bool)
            n130 = Or(x=w493, y=w490) -> (x .or. y?=w495:bool)
            n131 = And(x=w493, y=w492) -> (x .and. y?=w491:bool)
            n132 = case shown="True" w491 {
              tunnel: w494 -> [_ w498]
              frame False {
              }
              frame True {
                n133 = local write "New: Width"(w498) -> ()
              }
            }
            n134 = case shown="True" w495 {
              tunnel: w496 -> [w499 _]
              frame False {
                (unwired) 1
                n135 = local write "New: Width"(w499) -> ()
              }
              frame True {
                n136 = property on="New: Width" class="DigNum (strict)"("DisabledEnum"=0) -> ()  [unwired: 2 in, 2 out]
              }
            }
          }
          frame #2 {
            n137 = local read "Rec: Length"() -> (w506:dbl)
            n138 = case shown="True" w505 {
              tunnel: w506 -> [w514 _]
              frame False {
                n139 = local write "New: Length"(w514) -> ()
                n140 = property on="New: Length" class="DigNum (strict)"("DisabledEnum"=1) -> ()  [unwired: 2 in, 2 out]
              }
              frame True {
                n141 = property on="New: Length" class="DigNum (strict)"("DisabledEnum"=0) -> ()  [unwired: 2 in, 2 out]
              }
            }
            n142 = local read "Comments:"() -> (w503:string)
            n143 = local read "Rec: Dielectric (d)"() -> (w504:dbl)
            n144 = case shown="True" w501 {
              tunnel: w503 -> [w508 _]
              frame False {
                n145 = local write "New: Comments"(w508) -> ()
                n146 = property on="New: Comments" class="Str"("DisabledEnum"=1) -> ()  [unwired: 2 in, 2 out]
              }
              frame True {
                n147 = property on="New: Comments" class="Str"("DisabledEnum"=0) -> ()  [unwired: 2 in, 2 out]
              }
            }
            n148 = case shown="True" w502 {
              tunnel: w504 -> [w511 _]
              frame False {
                n149 = local write "New: Dielectric"(w511) -> ()
                n150 = property on="New: Dielectric" class="DigNum (strict)"("DisabledEnum"=1) -> ()  [unwired: 2 in, 2 out]
              }
              frame True {
                n151 = property on="New: Dielectric" class="DigNum (strict)"("DisabledEnum"=0) -> ()  [unwired: 2 in, 2 out]
              }
            }
          }
        }
        n152 = property on="Next File" class="Bool (strict)"("Value"=w45) -> (error out=w44:errorcluster)  [unwired: 2 in, 1 out]
        n153 = property on="Previous File" class="Bool (strict)"(error in=w44, "Value"=w45) -> (error out=w43:errorcluster)  [unwired: 1 in, 1 out]
        n154 = property on="Save" class="Bool (strict)"(error in=w43, "Value"=w45) -> (error out=w42:errorcluster)  [unwired: 1 in, 1 out]
        n155 = property on="Export" class="Bool (strict)"("Value"=w45) -> ()  [unwired: 2 in, 2 out]
        n156 = Unbundle By Name(w46) -> ()  [unwired: 8 out]
        n157 = property on="Save Next" class="Bool (strict)"(error in=w42, "Value"=w45) -> (error out=w41:errorcluster)  [unwired: 1 in, 1 out]
        n158 = property on="Discard" class="Bool (strict)"(error in=w41, "Value"=w45) -> (error out=w40:errorcluster)  [unwired: 1 in, 1 out]
        n159 = property on="Save Lines" class="Bool (strict)"(error in=w40, "Value"=w45) -> ()  [unwired: 1 in, 2 out]
        n160 = property on="Close" class="Bool (strict)"("Value"=w45) -> ()  [unwired: 2 in, 2 out]
        n161 = Cluster To Array(cluster=w46) -> (array=w57:bool[])
        n162 = call "Next State.vi"("Buttons []"=w57, "States []"=w58) -> ("Enum"=w49:T3)
        n163 = event shown="[7] \"Lin-Trans Slider\": Value Change" {
          selector: _ -> [_ _ _ _ _ _ _ _ _ _]
          dyn-events: _ -> [_ _ _ _ _ _ _ _ _ _]
          timeout: 5 -> [_ _ _ _ _ _ _ _ _ _]
          tunnel: w49 -> [w388 _ _ _ _ _ _ _ _ _]
          tunnel: [w388 MegaAwesome_States."Re-Calculated Values" MegaAwesome_States."Re-Calculated Values" MegaAwesome_States."Re-Calculated Values" MegaAwesome_States."Re-Calculated Values" MegaAwesome_States."Calculated Values" MegaAwesome_States."Re-Calculated Values" MegaAwesome_States."Re-Calculated Values" MegaAwesome_States."Re-Calculated Values" MegaAwesome_States."Re-Calculated Values"] -> w48
          event Timeout {
            n164 = event-data() -> ()  [unwired: 1 in, 2 out]
          }
          event "New: Dielectric": Value Change {
            n165 = event-data() -> ()  [unwired: 1 in, 5 out]
          }
          event "New: Length": Value Change {
            n166 = event-data() -> ()  [unwired: 1 in, 5 out]
          }
          event "New: Width": Value Change {
            n167 = event-data() -> ()  [unwired: 1 in, 5 out]
          }
          event "New: Temp": Value Change {
            n168 = event-data() -> ()  [unwired: 1 in, 5 out]
          }
          event "Num Pts Log", "Transport Style Controls", "Num Pts": Value Change {
            n169 = event-data() -> ()  [unwired: 1 in, 5 out]
          }
          event "Sat-Trans Slider": Value Change {
            n170 = event-data() -> ()  [unwired: 1 in, 5 out]
            n171 = local read "Sqrt-Sat"() -> (w417:cluster{dbl[], dbl[]}[])
            n172 = Decimate 1D Array(w417) -> (w401:cluster{dbl[], dbl[]}[], w402:cluster{dbl[], dbl[]}[])
            n173 = local read "Slider Min"() -> (w398:dbl)
            n174 = local read "Sat-Trans Slider"() -> (w396:dbl)
            n175 = Array To Cluster(array=w401) -> (cluster=w416:T22)
            n176 = local read "New: Dielectric"() -> (w411:dbl)
            n177 = local read "Num Pts"() -> (w394:dbl)
            n178 = local read "New: Width"() -> (w413:dbl)
            n179 = local read "New: Length"() -> (w412:dbl)
            n180 = Unbundle(w416) -> ("[0]"=w415:cluster{dbl[], dbl[]})  [unwired: 8 out]
            n181 = Absolute Value(x=w398) -> (abs(x)=w397:dbl)
            n182 = Unbundle(w415) -> (w399:dbl[], w414:dbl[])
            n183 = Add(x=w396, y=w397) -> (x+y=w395:dbl)
            n184 = Array Subset(array=w399, index=w395, length=w394) -> (w409:dbl[])
            n185 = local write "Sat Vg Array-Used"(w409) -> ()
            n186 = Array Subset(array=w414, index=w395, length=w394) -> (w410:dbl[])
            n187 = call "Mobility-Vt-Used Pts_Saturation.vi"("Width"=w413, "Length"=w412, "Dielectric (d)"=w411, "Sat Id Used"=w410, "Vg Used"=w409) -> ("Vt"=w405:dbl, "Mobility"=w406:dbl)  [unwired: 4 in, 1 out]
            n188 = local write "Index-Sat"(w395) -> ()
            n189 = local write "Sat Id-Used"(w410) -> ()
            n190 = Bundle(w409, w410) -> (w403:cluster{dbl[], dbl[]})  [unwired: 1 in]
            n191 = local read "Re-Calculated Values Cluster"() -> (w408:T10)
            n192 = Bundle By Name(cluster=w408, "Mobility-Sat"=w406, "Vt-Sat"=w405) -> (w407:T10)
            n193 = local write "Re-Calculated Values Cluster"(w407) -> ()
            n194 = Build Array (concatenate)(w401, w402, w403) -> (w400:cluster{dbl[], dbl[]}[])
            n195 = local write "Sqrt-Sat"(w400) -> ()
          }
          event "Lin-Trans Slider": Value Change {
            n196 = event-data() -> ()  [unwired: 1 in, 5 out]
            n197 = local read "Sqrt-Lin"() -> (w441:cluster{dbl[], dbl[]}[])
            n198 = Decimate 1D Array(w441) -> (w426:cluster{dbl[], dbl[]}[], w427:cluster{dbl[], dbl[]}[])
            n199 = local read "Slider Min"() -> (w423:dbl)
            n200 = Array To Cluster(array=w426) -> (cluster=w440:T22)
            n201 = local read "Lin-Trans Slider"() -> (w421:dbl)
            n202 = local read "New: Dielectric"() -> (w434:dbl)
            n203 = local read "Num Pts"() -> (w437:dbl)
            n204 = local read "New: Width"() -> (w436:dbl)
            n205 = local read "New: Length"() -> (w435:dbl)
            n206 = local read "Lin Vd"() -> (w418:dbl)
            n207 = Unbundle(w440) -> ("[0]"=w439:cluster{dbl[], dbl[]})  [unwired: 8 out]
            n208 = Absolute Value(x=w423) -> (abs(x)=w422:dbl)
            n209 = Unbundle(w439) -> (w424:dbl[], w438:dbl[])
            n210 = Add(x=w421, y=w422) -> (x+y=w420:dbl)
            n211 = Array Subset(array=w424, index=w420, length=w437) -> (w432:dbl[])
            n212 = local write "Lin-Vg Array-Used"(w432) -> ()
            n213 = Array Subset(array=w438, index=w420, length=w437) -> (w433:dbl[])
            n214 = call "Mobility-Vt-Used Pts_Linear.vi"("Width"=w436, "Length"=w435, "Vd"=w418, "Dielectric (d)"=w434, "Id Used"=w433, "Vg Used"=w432) -> ("Mobility"=w429:dbl)  [unwired: 3 in, 2 out]
            n215 = local write "Index-Lin"(w420) -> ()
            n216 = local write "Lin Id-Used"(w433) -> ()
            n217 = Bundle(w432, w433) -> (w428:cluster{dbl[], dbl[]})  [unwired: 1 in]
            n218 = local read "Re-Calculated Values Cluster"() -> (w431:T10)
            n219 = Bundle By Name(cluster=w431, "Moblitity-Lin"=w429) -> (w430:T10)
            n220 = local write "Re-Calculated Values Cluster"(w430) -> ()
            n221 = Build Array (concatenate)(w426, w427, w428) -> (w425:cluster{dbl[], dbl[]}[])
            n222 = local write "Sqrt-Lin"(w425) -> ()
          }
          event "Sat-Log Slider": Value Change {
            n223 = event-data() -> ()  [unwired: 1 in, 5 out]
            n224 = local read "Sat-Log"() -> (w444:cluster{dbl[], dbl[]}[])
            n225 = Decimate 1D Array(w444) -> (w451:cluster{dbl[], dbl[]}[], w452:cluster{dbl[], dbl[]}[])
            n226 = local read "Slider Min"() -> (w448:dbl)
            n227 = Array To Cluster(array=w451) -> (cluster=w461:T22)
            n228 = local read "Num Pts Log"() -> (w458:dbl)
            n229 = local read "Sat-Log Slider"() -> (w446:dbl)
            n230 = Unbundle(w461) -> ("[0]"=w460:cluster{dbl[], dbl[]})  [unwired: 8 out]
            n231 = Absolute Value(x=w448) -> (abs(x)=w447:dbl)
            n232 = Unbundle(w460) -> (w449:dbl[], w459:dbl[])
            n233 = Add(x=w446, y=w447) -> (x+y=w443:dbl)
            n234 = Array Subset(array=w449, index=w443, length=w458) -> (w456:dbl[])
            n235 = Array Subset(array=w459, index=w443, length=w458) -> (w457:dbl[])
            n236 = local write "Vg Array-Log-Used"(w456) -> ()
            n237 = local write "IndexLog-Sat"(w443) -> ()
            n238 = Bundle(w456, w457) -> (w442:cluster{dbl[], dbl[]})  [unwired: 1 in]
            n239 = call "STS-Used.vi"("Id Used"=w457, "Vg-Used"=w456) -> ("STS"=w453:dbl)  [unwired: 9 in]
            n240 = local write "Sat Id-Log-Used"(w457) -> ()
            n241 = local read "Re-Calculated Values Cluster"() -> (w455:T10)
            n242 = Bundle By Name(cluster=w455, "STS"=w453) -> (w454:T10)
            n243 = local write "Re-Calculated Values Cluster"(w454) -> ()
            n244 = Build Array (concatenate)(w451, w452, w442) -> (w450:cluster{dbl[], dbl[]}[])
            n245 = local write "Sat-Log"(w450) -> ()
          }
          event "Lin-Log Slider": Value Change {
            # "No Indicator for Lin-Log Slider Use"
            n246 = event-data() -> ()  [unwired: 1 in, 5 out]
            n247 = local read "Log-Lin"() -> (w465:cluster{dbl[], dbl[]}[])
            n248 = Decimate 1D Array(w465) -> (w471:cluster{dbl[], dbl[]}[], w472:cluster{dbl[], dbl[]}[])
            n249 = local read "Slider Min"() -> (w468:dbl)
            n250 = Array To Cluster(array=w471) -> (cluster=w478:T22)
            n251 = local read "Num Pts Log"() -> (w475:dbl)
            n252 = local read "Lin-Log Slider"() -> (w466:dbl)
            n253 = Unbundle(w478) -> ("[0]"=w477:cluster{dbl[], dbl[]})  [unwired: 8 out]
            n254 = Absolute Value(x=w468) -> (abs(x)=w467:dbl)
            n255 = Unbundle(w477) -> (w469:dbl[], w476:dbl[])
            n256 = Add(x=w466, y=w467) -> (x+y=w464:dbl)
            n257 = Array Subset(array=w469, index=w464, length=w475) -> (w473:dbl[])
            n258 = local write "Lin-Vg Array-Log Used"(w473) -> ()
            n259 = Array Subset(array=w476, index=w464, length=w475) -> (w474:dbl[])
            n260 = local write "IndexLog-Sat"(w464) -> ()
            n261 = Bundle(w473, w474) -> (w463:cluster{dbl[], dbl[]})  [unwired: 1 in]
            n262 = call "STS-Used.vi"("Id Used"=w474, "Vg-Used"=w473) -> ()  [unwired: 9 in, 1 out]
            n263 = local write "Lin Id-Log Used"(w474) -> ()
            n264 = Build Array (concatenate)(w471, w472, w463) -> (w470:cluster{dbl[], dbl[]}[])
            n265 = local write "Log-Lin"(w470) -> ()
          }
        }
      }
      frame "Read Data" {
        n266 = call "Recorded Values.vi"("Path"=w522) -> ("Recorded Char"=w540:T10, "Recorded Prop"=w530:T2, "Fabrication Prop"=w524:T5)  [unwired: 8 in]
        n267 = Strip Path(path=w522) -> (stripped path=w523:path, name=w521:string)
        n268 = local write "Fabrication Prop"(w524) -> ()
        n269 = local write "Recorded Prop"(w530) -> ()
        n270 = Unbundle By Name(w530) -> ("Date Recorded"=w529:string, "Index"=w527:string, "Length"=w528:dbl, "Width"=w526:dbl, "Sample Temp"=w525:dbl)
        n271 = local write "Recorded Values Cluster"(w540) -> ()
        n272 = Unbundle By Name(w530) -> ("Sample Temp"=w533:dbl)
        n273 = Unbundle By Name(w524) -> ("Dielectric (nm)"=w518:dbl, "Comments"=w517:string)
        n274 = List Folder(path=w523) -> (filenames=w519:string[])  [unwired: 3 in, 3 out]
        n275 = local write "Rec: Dielectric (d)"(w518) -> ()
        n276 = local write "Date Created"(w529) -> ()
        n277 = local write "Index"(w527) -> ()
        n278 = local write "Rec: Length"(w528) -> ()
        n279 = local write "Rec: Width"(w526) -> ()
        n280 = local write "Rec: Temp"(w525) -> ()
        n281 = Equal To 0?(x=w533) -> (x = 0?=w536:bool)
        n282 = Number To Decimal String(number=w533) -> (decimal integer string=w537:string)  [unwired: 1 in]
        n283 = local write "Comments:"(w517) -> ()
        n284 = Search 1D Array(1D array=w519, element=w521) -> (index of element=w516:i32)  [unwired: 1 in]
        n285 = Equal?(x="", y=w537) -> (x = y?=w535:bool)
        n286 = Index Array(array=w519, index=w516) -> (element=w520:string)
        n287 = Or(x=w536, y=w535) -> (x .or. y?=w534:bool)
        n288 = local write "Data Name:"(w520) -> ()
        n289 = case shown="False" w534 {
          tunnel: [w541 w542] -> w531
          tunnel: w533 -> [w541 _]
          frame False {
          }
          frame True {
            n290 = local read "Room Temp"() -> (w542:dbl)
          }
        }
        n291 = local write "New: Temp"(w531) -> ()
        n292 = Bundle By Name(cluster=w530, "Sample Temp"=w531) -> (w532:T2)
        n293 = local write "Recorded Prop"(w532) -> ()
      }
      frame "Calculated Values" {
        n294 = case shown="True" w543 {
          tunnel: w557 -> [_ w600]
          frame False {
          }
          frame True {
            n295 = local read "Transport Style Controls"() -> (w599:T11)
            n296 = call "TRF to TSP Plot.vi"("Transport Graph Properties"=w599, "Transfer File"=w600) -> ("Transport"=w598:cluster{ext[], ext[]}[])  [unwired: 7 in, 2 out]
            n297 = Array Size(array=w598) -> (size(s)=w597:i32)
            n298 = local write "Transport"(w598) -> ()
            n299 = for {
              N: w597 -> [_]
              tunnel: w599 -> [w604]
              i -> [w603]
              n300 = Unbundle By Name(w604) -> ("Transport Line Size"=w601:u16, "Transport Line Color"=w602:u32)
              n301 = property on="Transport" class="XYGraph (strict)"("Active Plot"=w603, "Plot.Plot Color"=w602, "Plot.Line Width"=w601) -> ()  [unwired: 2 in, 2 out]
            }
          }
        }
        n302 = local read "Fabrication Prop"() -> (w586:T5)
        n303 = local read "Recorded Prop"() -> (w579:T2)
        n304 = local read "Calculated Values Cluster"() -> (w596:T10)
        n305 = call "Mobility-Vt Calculator-File.vi"("NumPts"=w581, "Path"=w557) -> ("Used Points"=w574:T23, "Graph Cluster"=w563:T24, "Lin Vd"=w570:dbl, "Output"=w594:T25)  [unwired: 6 in]
        n306 = call "STS Calculator-File.vi"("NumPts"=w580, "Path"=w557) -> ("Used Points"=w568:T26, "XY Graph-Sat"=w550:cluster{dbl[], dbl[]}[], "XY Graph-Lin"=w551:cluster{dbl[], dbl[]}[], "Ouput"=w589:cluster{"STS-Sat":dbl, "STS-Lin":dbl})  [unwired: 6 in]
        n307 = Unbundle By Name(w586) -> ("Dielectric (nm)"=w584:dbl)
        n308 = Unbundle By Name(w579) -> ("Sample Temp"=w578:dbl)
        n309 = Unbundle By Name(w594) -> ("Mobility-Sat"=w593:dbl, "Vt-Sat"=w585:dbl, "Mobility-Lin"=w592:dbl, "Off I-Sat"=w591:dbl, "On/Off I-Sat"=w590:dbl)  [unwired: 1 out]
        n310 = local write "Lin Vd"(w570) -> ()
        n311 = Unbundle By Name(w589) -> ("STS-Sat"=w583:dbl)  [unwired: 1 out]
        n312 = local write "Sat-Log"(w550) -> ()
        n313 = local write "Log-Lin"(w551) -> ()
        n314 = call "Trap Density_VT.vi"("VT"=w585, "Dielectric"=w584) -> ("Trap Density-VT"=w588:dbl)
        n315 = call "Trap Density_STS.vi"("Temp (T) [K]"=w578, "S.T.S. (S)"=w583, "Dielectric"=w584) -> ("Trap Density (N)"=w587:dbl)  [unwired: 8 in]
        n316 = call "Image from TRF Display.vi"("No Image File"=w576, "Image Folder"=w577, "Transfer File"=w557) -> ("Image Out 2"=w544:T9, "Image Out"=w545:T9, "Image File"=w546:path, "Image Name"=w547:string)  [unwired: 5 in]
        n317 = Bundle By Name(cluster=w596, "Mobility-Sat"=w593, "Moblitity-Lin"=w592, "On/Off"=w590, "Off Current"=w591, "Vt-Sat"=w585, "STS"=w583, "Trap Density-VT"=w588, "Trap Density-STS"=w587) -> (w595:T10)
        n318 = Unbundle By Name(w568) -> ("Sat Vg Used"=w567:dbl[], "Sat Log(Id) Used"=w566:dbl[], "Lin Vg Used"=w565:dbl[], "Lin Log(Id) Used"=w564:dbl[], "STS Index-Sat"=w548:dbl, "STS Index-Lin"=w549:dbl)
        n319 = Unbundle By Name(w574) -> ("Sat Vg Used"=w573:dbl[], "Sat Sqrt(Id) Used"=w572:dbl[], "Lin Vg Used"=w571:dbl[], "Lin Sqrt(Id) Used"=w569:dbl[], "Index-Lin"=w559:dbl, "Index-Sat"=w558:dbl)
        n320 = local write "Image File"(w546) -> ()
        n321 = local write "Image Name"(w547) -> ()
        n322 = local write "Image Out"(w545) -> ()
        n323 = local write "Image Preview"(w544) -> ()
        n324 = local write "Vg Array-Log-Used"(w567) -> ()
        n325 = local write "Sat Id-Log-Used"(w566) -> ()
        n326 = local write "Lin-Vg Array-Log Used"(w565) -> ()
        n327 = local write "Lin Id-Log Used"(w564) -> ()
        n328 = local write "IndexLog-Sat"(w548) -> ()
        n329 = local write "Index-Lin"(w549) -> ()
        n330 = local write "Calculated Values Cluster"(w595) -> ()
        n331 = local write "Sat Vg Array-Used"(w573) -> ()
        n332 = local write "Sat Id-Used"(w572) -> ()
        n333 = local write "Lin-Vg Array-Used"(w571) -> ()
        n334 = local write "Lin Id-Used"(w569) -> ()
        n335 = local write "Index-Sat"(w558) -> ()
        n336 = local write "Index-Lin"(w559) -> ()
        n337 = local write "Lin-Log Slider"(w549) -> ()
        n338 = local write "Sat-Log Slider"(w548) -> ()
        n339 = local write "Sat-Trans Slider"(w558) -> ()
        n340 = local write "Lin-Trans Slider"(w559) -> ()
        n341 = Unbundle By Name(w563) -> ("Raw Sat"=w556:cluster{dbl[], dbl[]}[], "Sqrt Sat"=w560:cluster{dbl[], dbl[]}[], "Raw Lin"=w562:cluster{dbl[], dbl[]}[], "Sqrt Lin"=w561:cluster{dbl[], dbl[]}[])
        n342 = Index Array(array=w556) -> (element=w555:cluster{dbl[], dbl[]})  [unwired: 1 in]
        n343 = Unbundle(w555) -> (w554:dbl[])  [unwired: 1 out]
        n344 = Array Max & Min(array=w554) -> (max value=w553:dbl, min value=w552:dbl)  [unwired: 2 out]
        n345 = property on="Sat-Trans Slider" class="Slide (strict)"("Scale.Maximum"=w553, "Scale.Minimum"=w552) -> ()  [unwired: 2 in, 2 out]
        n346 = property on="Lin-Trans Slider" class="Slide (strict)"("Scale.Maximum"=w553, "Scale.Minimum"=w552) -> ()  [unwired: 2 in, 2 out]
        n347 = property on="Sat-Log Slider" class="Slide (strict)"("Scale.Maximum"=w553, "Scale.Minimum"=w552) -> ()  [unwired: 2 in, 2 out]
        n348 = property on="Lin-Log Slider" class="Slide (strict)"("Scale.Maximum"=w553, "Scale.Minimum"=w552) -> ()  [unwired: 2 in, 2 out]
        n349 = local write "Slider Max"(w553) -> ()
        n350 = local write "Slider Min"(w552) -> ()
        n351 = local write "Raw- Sat"(w556) -> ()
        n352 = local write "Raw- Lin"(w562) -> ()
        n353 = local write "Sqrt-Sat"(w560) -> ()
        n354 = local write "Sqrt-Lin"(w561) -> ()
      }
      frame "Re-Calculated Values" {
        n355 = local read "Vg Array-Log-Used"() -> (w613:dbl[])
        n356 = local read "Sat Vg Array-Used"() -> (w621:dbl[])
        n357 = local read "Lin-Vg Array-Used"() -> (w627:dbl[])
        n358 = local read "Sat Id-Log-Used"() -> (w612:dbl[])
        n359 = local read "New: Dielectric"() -> (w625:dbl)
        n360 = local read "New: Dielectric"() -> (w610:dbl)
        n361 = local read "New: Length"() -> (w624:dbl)
        n362 = local read "New: Length"() -> (w620:dbl)
        n363 = local read "New: Width"() -> (w623:dbl)
        n364 = local read "New: Width"() -> (w619:dbl)
        n365 = local read "Lin Id-Used"() -> (w626:dbl[])
        n366 = local read "Sat Id-Used"() -> (w618:dbl[])
        n367 = local read "Re-Calculated Values Cluster"() -> (w629:T10)
        n368 = local read "New: Dielectric"() -> (w609:dbl)
        n369 = local read "New: Temp"() -> (w608:dbl)
        n370 = local read "Lin Vd"() -> (w605:dbl)
        n371 = call "Mobility-Vt-Used Pts_Saturation.vi"("Width"=w619, "Length"=w620, "Dielectric (d)"=w610, "Sat Id Used"=w618, "Vg Used"=w621) -> ("Vt"=w616:dbl, "Mobility"=w617:dbl)  [unwired: 4 in, 1 out]
        n372 = call "STS-Used.vi"("Id Used"=w612, "Vg-Used"=w613) -> ("STS"=w611:dbl)  [unwired: 9 in]
        n373 = call "Mobility-Vt-Used Pts_Linear.vi"("Width"=w623, "Length"=w624, "Vd"=w605, "Dielectric (d)"=w625, "Id Used"=w626, "Vg Used"=w627) -> ("Mobility"=w622:dbl)  [unwired: 3 in, 2 out]
        n374 = call "Trap Density_VT.vi"("VT"=w616, "Dielectric"=w610) -> ("Trap Density-VT"=w615:dbl)
        n375 = call "Trap Density_STS.vi"("Temp (T) [K]"=w608, "S.T.S. (S)"=w611, "Dielectric"=w609) -> ("Trap Density (N)"=w607:dbl)  [unwired: 8 in]
        n376 = Bundle By Name(cluster=w629, "Mobility-Sat"=w617, "Moblitity-Lin"=w622, "Vt-Sat"=w616, "STS"=w611, "Trap Density-VT"=w615, "Trap Density-STS"=w607) -> (w628:T10)
        n377 = local write "Re-Calculated Values Cluster"(w628) -> ()
      }
      frame "Next File" {
        n378 = Strip Path(path=w646) -> (stripped path=w636:path, name=w644:string)
        n379 = local write "Transfer Folder"(w636) -> ()
        n380 = List Folder(path=w636) -> (filenames=w630:string[], error out=w639:errorcluster)  [unwired: 3 in, 2 out]
        n381 = Array Size(array=w630) -> (size(s)=w643:i32)
        n382 = Search 1D Array(1D array=w630, element=w644) -> (index of element=w641:i32)  [unwired: 1 in]
        n383 = Decrement(x=w643) -> (x-1=w642:i32)
        n384 = Equal?(x=w642, y=w641) -> (x = y?=w640:bool)
        n385 = case shown="False" w640 {
          tunnel: w632 -> [w649 _]
          tunnel: [w648 0] -> w631
          tunnel: w639 -> [w647 w650]
          tunnel: [w647 w650] -> _
          frame False {
            n386 = Increment(x=w649) -> (x+1=w648:i32)
          }
          frame True {
          }
        }
        n387 = Path To String(path=w636) -> (string=w637:string)
        n388 = Index Array(array=w630, index=w631) -> (element=w638:string)
        n389 = Concatenate Strings(w637, "\\", w638) -> (w634:string)
        n390 = String To Path(string=w634) -> (path=w633:path)
        n391 = local write "Transfer File"(w633) -> ()
      }
      frame "Previous File" {
        n392 = Strip Path(path=w658) -> (stripped path=w655:path, name=w667:string)
        n393 = local write "Transfer Folder"(w655) -> ()
        n394 = List Folder(path=w655) -> (filenames=w659:string[], error out=w664:errorcluster)  [unwired: 3 in, 2 out]
        n395 = Array Size(array=w659) -> (size(s)=w653:i32)
        n396 = Search 1D Array(1D array=w659, element=w667) -> (index of element=w666:i32)  [unwired: 1 in]
        n397 = Decrement(x=w653) -> (x-1=w652:i32)
        n398 = Equal To 0?(x=w666) -> (x = 0?=w665:bool)
        n399 = case shown="False" w665 {
          tunnel: w657 -> [w671 _]
          tunnel: [w670 w672] -> w656
          tunnel: w664 -> [w669 w673]
          tunnel: [w669 w673] -> _
          tunnel: w652 -> [_ w672]
          frame False {
            n400 = Decrement(x=w671) -> (x-1=w670:i32)
          }
          frame True {
          }
        }
        n401 = Path To String(path=w655) -> (string=w654:string)
        n402 = Index Array(array=w659, index=w656) -> (element=w663:string)
        n403 = Concatenate Strings(w654, "\\", w663) -> (w661:string)
        n404 = String To Path(string=w661) -> (path=w660:path)
        n405 = local write "Transfer File"(w660) -> ()
      }
      frame "Discard File" {
      }
      frame "Save" {
        n406 = stacked-sequence {
          seq-local: [w691 _] -> [_ w1188]
          seq-local: [w690 _] -> [_ w1186]
          tunnel: w682 -> [w692 w1189]
          frame #0 {
            # "Saves each Re-calculated parameter in sequence"
            n407 = stacked-sequence {
              tunnel: [_ _ _ _ _ _ _ _ _ _ _ _ _ w1156] -> w690
              tunnel: w692 -> [w712 _ _ _ _ _ _ _ _ _ _ _ _ _]
              frame #0 {
                n408 = call-poly <vilib>:"Read From Spreadsheet File.vi"("file path (dialog if empty)"=w712) -> ("all rows"=w711:string[][])  [unwired: 6 in, 4 out]
                n409 = Array Size(array=w711) -> (size(s)=w716:i32[])
                n410 = Array Subset(array=w711, index (row)=0, index (col)=0, length (col)=3) -> (w720:string[][])  [unwired: 1 in]
                n411 = Index Array(array=w716, index=0) -> (element=w714:i32)
                n412 = Reshape Array(w720, w714) -> (w713:string[])
                n413 = Search 1D Array(1D array=w713, element="Dielectric (nm):") -> (index of element=w723:i32)  [unwired: 1 in]
                n414 = Equal?(x=w723, y=-1) -> (x = y?=w722:bool)
                n415 = case shown="False" w722 {
                  tunnel: w711 -> [w731 w735]
                  tunnel: w723 -> [w727 _]
                  tunnel: [w726 w735] -> w721
                  frame False {
                    n416 = local read "Rec: Dielectric (d)"() -> (w733:dbl)
                    n417 = Number To Fractional String(number=w733) -> (F-format string=w728:string)  [unwired: 3 in]
                    n418 = Divide(x=w727, y=3) -> (x/y=w730:dbl)
                    n419 = To Word Integer(number=w730) -> (16bit integer=w729:i16)
                    n420 = Replace Array Subset(array=w731, new element=w728, index (row)=w729, index (col)=1) -> (w726:string[][])
                  }
                  frame True {
                  }
                }
                n421 = local write "Save Array"(w721) -> ()
              }
              frame #1 {
                n422 = local read "Save Array"() -> (w737:string[][])
                n423 = Array Size(array=w737) -> (size(s)=w740:i32[])
                n424 = Array Subset(array=w737, index (row)=0, index (col)=0, length (col)=3) -> (w744:string[][])  [unwired: 1 in]
                n425 = Index Array(array=w740, index=0) -> (element=w738:i32)
                n426 = Reshape Array(w744, w738) -> (w736:string[])
                n427 = Search 1D Array(1D array=w736, element="Comments:") -> (index of element=w747:i32)  [unwired: 1 in]
                n428 = Equal?(x=w747, y=-1) -> (x = y?=w746:bool)
                n429 = case shown="False" w746 {
                  tunnel: w737 -> [w755 w758]
                  tunnel: w747 -> [w752 _]
                  tunnel: [w751 w758] -> w745
                  frame False {
                    n430 = local read "New: Comments"() -> (w750:string)
                    n431 = Divide(x=w752, y=3) -> (x/y=w754:dbl)
                    n432 = To Word Integer(number=w754) -> (16bit integer=w753:i16)
                    n433 = Replace Array Subset(array=w755, new element=w750, index (row)=w753, index (col)=1) -> (w751:string[][])
                  }
                  frame True {
                  }
                }
                n434 = local write "Save Array"(w745) -> ()
              }
              frame #2 {
                n435 = local read "Save Array"() -> (w760:string[][])
                n436 = Array Size(array=w760) -> (size(s)=w763:i32[])
                n437 = Array Subset(array=w760, index (row)=0, index (col)=0, length (col)=3) -> (w767:string[][])  [unwired: 1 in]
                n438 = Index Array(array=w763, index=0) -> (element=w761:i32)
                n439 = Reshape Array(w767, w761) -> (w759:string[])
                n440 = Search 1D Array(1D array=w759, element="Length (um):") -> (index of element=w770:i32)  [unwired: 1 in]
                n441 = Equal?(x=w770, y=-1) -> (x = y?=w769:bool)
                n442 = case shown="False" w769 {
                  tunnel: w760 -> [w780 w783]
                  tunnel: w770 -> [w777 _]
                  tunnel: [w776 w783] -> w768
                  frame False {
                    n443 = local read "New: Length"() -> (w773:dbl)
                    n444 = Divide(x=w777, y=3) -> (x/y=w779:dbl)
                    n445 = Format Value(format string="%#g", value (0)=w773) -> (output string=w774:string)  [unwired: 1 in]
                    n446 = To Word Integer(number=w779) -> (16bit integer=w778:i16)
                    n447 = Replace Array Subset(array=w780, new element=w774, index (row)=w778, index (col)=1) -> (w776:string[][])
                  }
                  frame True {
                  }
                }
                n448 = local write "Save Array"(w768) -> ()
              }
              frame #3 {
                n449 = local read "Save Array"() -> (w785:string[][])
                n450 = Array Size(array=w785) -> (size(s)=w790:i32[])
                n451 = Array Subset(array=w785, index (row)=0, index (col)=0, length (col)=3) -> (w786:string[][])  [unwired: 1 in]
                n452 = Index Array(array=w790, index=0) -> (element=w792:i32)
                n453 = Reshape Array(w786, w792) -> (w784:string[])
                n454 = Search 1D Array(1D array=w784, element="Width (um):") -> (index of element=w795:i32)  [unwired: 1 in]
                n455 = Equal?(x=w795, y=-1) -> (x = y?=w794:bool)
                n456 = case shown="False" w794 {
                  tunnel: w795 -> [w803 _]
                  tunnel: w785 -> [w802 w808]
                  tunnel: [w801 w808] -> w793
                  frame False {
                    n457 = local read "New: Width"() -> (w798:dbl)
                    n458 = Divide(x=w803, y=3) -> (x/y=w805:dbl)
                    n459 = To Word Integer(number=w805) -> (16bit integer=w804:i16)
                    n460 = Format Value(format string="%#g", value (0)=w798) -> (output string=w799:string)  [unwired: 1 in]
                    n461 = Replace Array Subset(array=w802, new element=w799, index (row)=w804, index (col)=1) -> (w801:string[][])
                  }
                  frame True {
                  }
                }
                n462 = local write "Save Array"(w793) -> ()
              }
              frame #4 {
                w818 = "Sample Temp (K):"
                n463 = local read "Save Array"() -> (w810:string[][])
                n464 = Array Size(array=w810) -> (size(s)=w815:i32[])
                n465 = Array Subset(array=w810, index (row)=0, index (col)=0, length (col)=3) -> (w811:string[][])  [unwired: 1 in]
                n466 = Index Array(array=w815, index=0) -> (element=w817:i32)
                n467 = Reshape Array(w811, w817) -> (w809:string[])
                n468 = Search 1D Array(1D array=w809, element=w818) -> (index of element=w821:i32)  [unwired: 1 in]
                n469 = Equal?(x=w821, y=-1) -> (x = y?=w820:bool)
                n470 = case shown="False" w820 {
                  tunnel: w810 -> [w830 w844]
                  tunnel: w821 -> [w827 _]
                  tunnel: [w826 w843] -> w819
                  tunnel: w809 -> [_ w846]
                  tunnel: w818 -> [_ w833]
                  frame False {
                    n471 = local read "New: Temp"() -> (w824:dbl)
                    n472 = Divide(x=w827, y=3) -> (x/y=w829:dbl)
                    n473 = Format Value(format string="%#g", value (0)=w824) -> (output string=w823:string)  [unwired: 1 in]
                    n474 = To Word Integer(number=w829) -> (16bit integer=w828:i16)
                    n475 = Replace Array Subset(array=w830, new element=w823, index (row)=w828, index (col)=1) -> (w826:string[][])
                  }
                  frame True {
                    n476 = local read "New: Temp"() -> (w835:dbl)
                    n477 = Search 1D Array(1D array=w846, element="Width (um):") -> (index of element=w840:i32)  [unwired: 1 in]
                    n478 = Divide(x=w840, y=3) -> (x/y=w841:dbl)
                    n479 = To Word Integer(number=w841) -> (16bit integer=w839:i16)
                    n480 = Format Value(format string="%#g", value (0)=w835) -> (output string=w834:string)  [unwired: 1 in]
                    n481 = Build Array(w833, w834) -> (w837:string[])
                    n482 = Increment(x=w839) -> (x+1=w838:i16)
                    n483 = Insert Into Array(array=w844, index (row)=w838, new element=w837) -> (w843:string[][])  [unwired: 1 in]
                  }
                }
                n484 = local write "Save Array"(w819) -> ()
              }
              frame #5 {
                w856 = "Mobility-Sat (cm^2/Vs):"
                n485 = local read "Save Array"() -> (w848:string[][])
                n486 = Array Size(array=w848) -> (size(s)=w853:i32[])
                n487 = Array Subset(array=w848, index (row)=0, index (col)=0, length (col)=3) -> (w849:string[][])  [unwired: 1 in]
                n488 = Index Array(array=w853, index=0) -> (element=w855:i32)
                n489 = Reshape Array(w849, w855) -> (w847:string[])
                n490 = Search 1D Array(1D array=w847, element=w856) -> (index of element=w859:i32)  [unwired: 1 in]
                n491 = Equal?(x=w859, y=-1) -> (x = y?=w858:bool)
                n492 = case shown="False" w858 {
                  tunnel: w848 -> [w869 w879]
                  tunnel: w859 -> [w866 _]
                  tunnel: [w865 w878] -> w857
                  tunnel: w847 -> [_ w876]
                  tunnel: w856 -> [_ w874]
                  frame False {
                    n493 = local read "Re-Calculated Values Cluster"() -> (w862:T10)
                    n494 = Unbundle By Name(w862) -> ("Mobility-Sat"=w861:dbl)
                    n495 = Divide(x=w866, y=3) -> (x/y=w868:dbl)
                    n496 = To Word Integer(number=w868) -> (16bit integer=w867:i16)
                    n497 = Format Value(format string="%#g", value (0)=w861) -> (output string=w863:string)  [unwired: 1 in]
                    n498 = Replace Array Subset(array=w869, new element=w863, index (row)=w867, index (col)=1) -> (w865:string[][])
                  }
                  frame True {
                    n499 = local read "Re-Calculated Values Cluster"() -> (w873:T10)
                    n500 = Unbundle By Name(w873) -> ("Mobility-Sat"=w872:dbl)
                    n501 = Search 1D Array(1D array=w876, element="Mobility (cm^2/Vs):") -> (index of element=w882:i32)  [unwired: 1 in]
                    n502 = Divide(x=w882, y=3) -> (x/y=w883:dbl)
                    n503 = To Word Integer(number=w883) -> (16bit integer=w875:i16)
                    n504 = Format Value(format string="%#g", value (0)=w872) -> (output string=w877:string)  [unwired: 1 in]
                    n505 = Build Array(w874, w877) -> (w881:string[])
                    n506 = Replace Array Subset(array=w879, new element=w881, index (row)=w875) -> (w878:string[][])  [unwired: 1 in]
                  }
                }
                n507 = local write "Save Array"(w857) -> ()
              }
              frame #6 {
                w895 = "Mobility-Lin (cm^2/Vs):"
                n508 = local read "Save Array"() -> (w886:string[][])
                n509 = Array Size(array=w886) -> (size(s)=w892:i32[])
                n510 = Array Subset(array=w886, index (row)=0, index (col)=0, length (col)=3) -> (w888:string[][])  [unwired: 1 in]
                n511 = Index Array(array=w892, index=0) -> (element=w894:i32)
                n512 = Reshape Array(w888, w894) -> (w887:string[])
                n513 = Search 1D Array(1D array=w887, element=w895) -> (index of element=w898:i32)  [unwired: 1 in]
                n514 = Equal?(x=w898, y=-1) -> (x = y?=w897:bool)
                n515 = case shown="True" w897 {
                  tunnel: w886 -> [w908 w916]
                  tunnel: w898 -> [w905 _]
                  tunnel: [w904 w915] -> w896
                  tunnel: w887 -> [_ w914]
                  tunnel: w895 -> [_ w913]
                  frame False {
                    n516 = local read "Re-Calculated Values Cluster"() -> (w901:T10)
                    n517 = Unbundle By Name(w901) -> ("Moblitity-Lin"=w900:dbl)
                    n518 = Divide(x=w905, y=3) -> (x/y=w907:dbl)
                    n519 = To Word Integer(number=w907) -> (16bit integer=w906:i16)
                    n520 = Format Value(format string="%#g", value (0)=w900) -> (output string=w902:string)  [unwired: 1 in]
                    n521 = Replace Array Subset(array=w908, new element=w902, index (row)=w906, index (col)=1) -> (w904:string[][])
                  }
                  frame True {
                    n522 = local read "Re-Calculated Values Cluster"() -> (w912:T10)
                    n523 = Unbundle By Name(w912) -> ("Moblitity-Lin"=w911:dbl)
                    n524 = Search 1D Array(1D array=w914, element="Mobility-Sat (cm^2/Vs):") -> (index of element=w921:i32)  [unwired: 1 in]
                    n525 = Divide(x=w921, y=3) -> (x/y=w922:dbl)
                    n526 = To Word Integer(number=w922) -> (16bit integer=w920:i16)
                    n527 = Format Value(format string="%#g", value (0)=w911) -> (output string=w925:string)  [unwired: 1 in]
                    n528 = Build Array(w913, w925) -> (w918:string[])
                    n529 = Increment(x=w920) -> (x+1=w919:i16)
                    n530 = Insert Into Array(array=w916, index (row)=w919, new element=w918) -> (w915:string[][])  [unwired: 1 in]
                  }
                }
                n531 = local write "Save Array"(w896) -> ()
              }
              frame #7 {
                w935 = "On/Off I-Sat:"
                n532 = local read "Save Array"() -> (w926:string[][])
                n533 = Array Size(array=w926) -> (size(s)=w932:i32[])
                n534 = Array Subset(array=w926, index (row)=0, index (col)=0, length (col)=3) -> (w928:string[][])  [unwired: 1 in]
                n535 = Index Array(array=w932, index=0) -> (element=w934:i32)
                n536 = Reshape Array(w928, w934) -> (w927:string[])
                n537 = Search 1D Array(1D array=w927, element=w935) -> (index of element=w938:i32)  [unwired: 1 in]
                n538 = Equal?(x=w938, y=-1) -> (x = y?=w937:bool)
                n539 = case shown="True" w937 {
                  tunnel: w926 -> [w948 w957]
                  tunnel: w938 -> [w945 _]
                  tunnel: [w944 w958] -> w936
                  tunnel: w927 -> [_ w955]
                  tunnel: w935 -> [_ w953]
                  frame False {
                    n540 = local read "Re-Calculated Values Cluster"() -> (w941:T10)
                    n541 = Divide(x=w945, y=3) -> (x/y=w947:dbl)
                    n542 = Unbundle By Name(w941) -> ("On/Off"=w940:dbl)
                    n543 = To Word Integer(number=w947) -> (16bit integer=w946:i16)
                    n544 = Format Value(format string="%#g", value (0)=w940) -> (output string=w942:string)  [unwired: 1 in]
                    n545 = Replace Array Subset(array=w948, new element=w942, index (row)=w946, index (col)=1) -> (w944:string[][])
                  }
                  frame True {
                    n546 = local read "Re-Calculated Values Cluster"() -> (w952:T10)
                    n547 = Unbundle By Name(w952) -> ("On/Off"=w951:dbl)
                    n548 = Search 1D Array(1D array=w955, element="On/Off Current:") -> (index of element=w961:i32)  [unwired: 1 in]
                    n549 = Divide(x=w961, y=3) -> (x/y=w962:dbl)
                    n550 = To Word Integer(number=w962) -> (16bit integer=w954:i16)
                    n551 = Format Value(format string="%#g", value (0)=w951) -> (output string=w956:string)  [unwired: 1 in]
                    n552 = Build Array(w953, w956) -> (w960:string[])
                    n553 = Replace Array Subset(array=w957, new element=w960, index (row)=w954) -> (w958:string[][])  [unwired: 1 in]
                  }
                }
                n554 = local write "Save Array"(w936) -> ()
              }
              frame #8 {
                w974 = "Off I-Sat (A):"
                n555 = local read "Save Array"() -> (w965:string[][])
                n556 = Array Size(array=w965) -> (size(s)=w971:i32[])
                n557 = Array Subset(array=w965, index (row)=0, index (col)=0, length (col)=3) -> (w967:string[][])  [unwired: 1 in]
                n558 = Index Array(array=w971, index=0) -> (element=w973:i32)
                n559 = Reshape Array(w967, w973) -> (w966:string[])
                n560 = Search 1D Array(1D array=w966, element=w974) -> (index of element=w977:i32)  [unwired: 1 in]
                n561 = Equal?(x=w977, y=-1) -> (x = y?=w976:bool)
                n562 = case shown="True" w976 {
                  tunnel: w965 -> [w987 w995]
                  tunnel: w977 -> [w984 _]
                  tunnel: [w983 w994] -> w975
                  tunnel: w966 -> [_ w993]
                  tunnel: w974 -> [_ w992]
                  frame False {
                    n563 = local read "Re-Calculated Values Cluster"() -> (w980:T10)
                    n564 = Unbundle By Name(w980) -> ("Off Current"=w979:dbl)
                    n565 = Divide(x=w984, y=3) -> (x/y=w986:dbl)
                    n566 = Format Value(format string="%#g", value (0)=w979) -> (output string=w981:string)  [unwired: 1 in]
                    n567 = To Word Integer(number=w986) -> (16bit integer=w985:i16)
                    n568 = Replace Array Subset(array=w987, new element=w981, index (row)=w985, index (col)=1) -> (w983:string[][])
                  }
                  frame True {
                    n569 = local read "Re-Calculated Values Cluster"() -> (w991:T10)
                    n570 = Unbundle By Name(w991) -> ("Off Current"=w990:dbl)
                    n571 = Search 1D Array(1D array=w993, element="On/Off I-Sat:") -> (index of element=w1000:i32)  [unwired: 1 in]
                    n572 = Divide(x=w1000, y=3) -> (x/y=w1001:dbl)
                    n573 = To Word Integer(number=w1001) -> (16bit integer=w999:i16)
                    n574 = Format Value(format string="%#g", value (0)=w990) -> (output string=w1004:string)  [unwired: 1 in]
                    n575 = Build Array(w992, w1004) -> (w997:string[])
                    n576 = Increment(x=w999) -> (x+1=w998:i16)
                    n577 = Insert Into Array(array=w995, index (row)=w998, new element=w997) -> (w994:string[][])  [unwired: 1 in]
                  }
                }
                n578 = local write "Save Array"(w975) -> ()
              }
              frame #9 {
                w1006 = "Vt-Sat (V):"
                n579 = local read "Save Array"() -> (w1007:string[][])
                n580 = Array Size(array=w1007) -> (size(s)=w1012:i32[])
                n581 = Array Subset(array=w1007, index (row)=0, index (col)=0, length (col)=3) -> (w1008:string[][])  [unwired: 1 in]
                n582 = Index Array(array=w1012, index=0) -> (element=w1014:i32)
                n583 = Reshape Array(w1008, w1014) -> (w1005:string[])
                n584 = Search 1D Array(1D array=w1005, element=w1006) -> (index of element=w1017:i32)  [unwired: 1 in]
                n585 = Equal?(x=w1017, y=-1) -> (x = y?=w1016:bool)
                n586 = case shown="False" w1016 {
                  tunnel: w1007 -> [w1026 w1036]
                  tunnel: w1017 -> [w1022 _]
                  tunnel: [w1021 w1035] -> w1015
                  tunnel: w1006 -> [_ w1034]
                  tunnel: w1005 -> [_ w1033]
                  frame False {
                    n587 = local read "Re-Calculated Values Cluster"() -> (w1020:T10)
                    n588 = Unbundle By Name(w1020) -> ("Vt-Sat"=w1019:dbl)
                    n589 = Divide(x=w1022, y=3) -> (x/y=w1025:dbl)
                    n590 = To Word Integer(number=w1025) -> (16bit integer=w1024:i16)
                    n591 = Number To Fractional String(number=w1019) -> (F-format string=w1023:string)  [unwired: 3 in]
                    n592 = Replace Array Subset(array=w1026, new element=w1023, index (row)=w1024, index (col)=1) -> (w1021:string[][])
                  }
                  frame True {
                    n593 = local read "Re-Calculated Values Cluster"() -> (w1030:T10)
                    n594 = Unbundle By Name(w1030) -> ("Vt-Sat"=w1029:dbl)
                    n595 = Search 1D Array(1D array=w1033, element="Threshold V (V):") -> (index of element=w1032:i32)  [unwired: 1 in]
                    n596 = Divide(x=w1032, y=3) -> (x/y=w1039:dbl)
                    n597 = To Word Integer(number=w1039) -> (16bit integer=w1031:i16)
                    n598 = Format Value(format string="%#g", value (0)=w1029) -> (output string=w1042:string)  [unwired: 1 in]
                    n599 = Build Array(w1034, w1042) -> (w1038:string[])
                    n600 = Replace Array Subset(array=w1036, new element=w1038, index (row)=w1031) -> (w1035:string[][])  [unwired: 1 in]
                  }
                }
                n601 = local write "Save Array"(w1015) -> ()
              }
              frame #10 {
                n602 = disable-structure shown="Disabled" {
                  frame Disabled {
                    n603 = local read "Save Array"() -> (w1043:string[][])
                    n604 = Array Size(array=w1043) -> (size(s)=w1049:i32[])
                    n605 = Array Subset(array=w1043, index (row)=0, index (col)=0, length (col)=3) -> (w1045:string[][])  [unwired: 1 in]
                    n606 = Index Array(array=w1049, index=0) -> (element=w1051:i32)
                    n607 = Reshape Array(w1045, w1051) -> (w1044:string[])
                    n608 = Search 1D Array(1D array=w1044, element="VT-Lin (V):") -> (index of element=w1054:i32)  [unwired: 1 in]
                    n609 = Equal?(x=w1054, y=-1) -> (x = y?=w1053:bool)
                    n610 = case shown="False" w1053 {
                      tunnel: w1043 -> [w1063 w1066]
                      tunnel: w1054 -> [w1060 _]
                      tunnel: [w1059 w1066] -> w1052
                      frame False {
                        n611 = Divide(x=w1060, y=3) -> (x/y=w1062:dbl)
                        n612 = To Word Integer(number=w1062) -> (16bit integer=w1061:i16)
                        n613 = Format Value(format string="%#g") -> (output string=w1057:string)  [unwired: 2 in]
                        n614 = Replace Array Subset(array=w1063, new element=w1057, index (row)=w1061, index (col)=1) -> (w1059:string[][])
                      }
                      frame True {
                      }
                    }
                    n615 = local write "Save Array"(w1052) -> ()
                  }
                  frame Enabled {
                  }
                }
              }
              frame #11 {
                w1067 = "STS-Sat (V/decade):"
                n616 = local read "Save Array"() -> (w1069:string[][])
                n617 = Array Size(array=w1069) -> (size(s)=w1074:i32[])
                n618 = Array Subset(array=w1069, index (row)=0, index (col)=0, length (col)=3) -> (w1070:string[][])  [unwired: 1 in]
                n619 = Index Array(array=w1074, index=0) -> (element=w1076:i32)
                n620 = Reshape Array(w1070, w1076) -> (w1068:string[])
                n621 = Search 1D Array(1D array=w1068, element=w1067) -> (index of element=w1079:i32)  [unwired: 1 in]
                n622 = Equal?(x=w1079, y=-1) -> (x = y?=w1078:bool)
                n623 = case shown="True" w1078 {
                  tunnel: w1069 -> [w1089 w1097]
                  tunnel: w1079 -> [w1086 _]
                  tunnel: [w1085 w1098] -> w1077
                  tunnel: w1068 -> [_ w1096]
                  tunnel: w1067 -> [_ w1095]
                  frame False {
                    n624 = local read "Re-Calculated Values Cluster"() -> (w1081:T10)
                    n625 = Unbundle By Name(w1081) -> ("STS"=w1082:dbl)
                    n626 = Divide(x=w1086, y=3) -> (x/y=w1088:dbl)
                    n627 = To Word Integer(number=w1088) -> (16bit integer=w1087:i16)
                    n628 = Format Value(format string="%#g", value (0)=w1082) -> (output string=w1083:string)  [unwired: 1 in]
                    n629 = Replace Array Subset(array=w1089, new element=w1083, index (row)=w1087, index (col)=1) -> (w1085:string[][])
                  }
                  frame True {
                    n630 = local read "Re-Calculated Values Cluster"() -> (w1092:T10)
                    n631 = Unbundle By Name(w1092) -> ("STS"=w1093:dbl)
                    n632 = Search 1D Array(1D array=w1096, element="S.T.S. (V/decade):") -> (index of element=w1101:i32)  [unwired: 1 in]
                    n633 = Divide(x=w1101, y=3) -> (x/y=w1102:dbl)
                    n634 = To Word Integer(number=w1102) -> (16bit integer=w1094:i16)
                    n635 = Format Value(format string="%#g", value (0)=w1093) -> (output string=w1105:string)  [unwired: 1 in]
                    n636 = Build Array(w1095, w1105) -> (w1100:string[])
                    n637 = Replace Array Subset(array=w1097, new element=w1100, index (row)=w1094) -> (w1098:string[][])  [unwired: 1 in]
                  }
                }
                n638 = local write "Save Array"(w1077) -> ()
              }
              frame #12 {
                w1106 = "Trap Density-VT (Traps/Vcm^2):"
                n639 = local read "Save Array"() -> (w1108:string[][])
                n640 = Array Size(array=w1108) -> (size(s)=w1113:i32[])
                n641 = Array Subset(array=w1108, index (row)=0, index (col)=0, length (col)=3) -> (w1109:string[][])  [unwired: 1 in]
                n642 = Index Array(array=w1113, index=0) -> (element=w1115:i32)
                n643 = Reshape Array(w1109, w1115) -> (w1107:string[])
                n644 = Search 1D Array(1D array=w1107, element=w1106) -> (index of element=w1118:i32)  [unwired: 1 in]
                n645 = Equal?(x=w1118, y=-1) -> (x = y?=w1117:bool)
                n646 = case shown="True" w1117 {
                  tunnel: w1108 -> [w1128 w1135]
                  tunnel: w1118 -> [w1124 _]
                  tunnel: [w1123 w1136] -> w1116
                  tunnel: w1107 -> [_ w1134]
                  tunnel: w1106 -> [_ w1133]
                  frame False {
                    n647 = local read "Re-Calculated Values Cluster"() -> (w1121:T10)
                    n648 = Unbundle By Name(w1121) -> ("Trap Density-VT"=w1120:dbl)
                    n649 = Divide(x=w1124, y=3) -> (x/y=w1127:dbl)
                    n650 = To Word Integer(number=w1127) -> (16bit integer=w1126:i16)
                    n651 = Format Value(format string="%#g", value (0)=w1120) -> (output string=w1125:string)  [unwired: 1 in]
                    n652 = Replace Array Subset(array=w1128, new element=w1125, index (row)=w1126, index (col)=1) -> (w1123:string[][])
                  }
                  frame True {
                    n653 = local read "Re-Calculated Values Cluster"() -> (w1132:T10)
                    n654 = Unbundle By Name(w1132) -> ("Trap Density-VT"=w1131:dbl)
                    n655 = Search 1D Array(1D array=w1134, element="STS-Sat (V/decade):") -> (index of element=w1141:i32)  [unwired: 1 in]
                    n656 = Divide(x=w1141, y=3) -> (x/y=w1140:dbl)
                    n657 = To Word Integer(number=w1140) -> (16bit integer=w1142:i16)
                    n658 = Format Value(format string="%#g", value (0)=w1131) -> (output string=w1137:string)  [unwired: 1 in]
                    n659 = Build Array(w1133, w1137) -> (w1144:string[])
                    n660 = Increment(x=w1142) -> (x+1=w1143:i16)
                    n661 = Insert Into Array(array=w1135, index (row)=w1143, new element=w1144) -> (w1136:string[][])  [unwired: 1 in]
                  }
                }
                n662 = local write "Save Array"(w1116) -> ()
              }
              frame #13 {
                w1146 = "Trap Density-STS (Traps/Vcm^2):"
                n663 = local read "Save Array"() -> (w1148:string[][])
                n664 = Array Size(array=w1148) -> (size(s)=w1153:i32[])
                n665 = Array Subset(array=w1148, index (row)=0, index (col)=0, length (col)=3) -> (w1149:string[][])  [unwired: 1 in]
                n666 = Index Array(array=w1153, index=0) -> (element=w1155:i32)
                n667 = Reshape Array(w1149, w1155) -> (w1147:string[])
                n668 = Search 1D Array(1D array=w1147, element=w1146) -> (index of element=w1158:i32)  [unwired: 1 in]
                n669 = Equal?(x=w1158, y=-1) -> (x = y?=w1157:bool)
                n670 = case shown="True" w1157 {
                  tunnel: w1148 -> [w1168 w1175]
                  tunnel: w1158 -> [w1165 _]
                  tunnel: [w1164 w1176] -> w1156
                  tunnel: w1147 -> [_ w1174]
                  tunnel: w1146 -> [_ w1173]
                  frame False {
                    n671 = local read "Re-Calculated Values Cluster"() -> (w1161:T10)
                    n672 = Unbundle By Name(w1161) -> ("Trap Density-STS"=w1160:dbl)
                    n673 = Divide(x=w1165, y=3) -> (x/y=w1167:dbl)
                    n674 = To Word Integer(number=w1167) -> (16bit integer=w1166:i16)
                    n675 = Format Value(format string="%#g", value (0)=w1160) -> (output string=w1162:string)  [unwired: 1 in]
                    n676 = Replace Array Subset(array=w1168, new element=w1162, index (row)=w1166, index (col)=1) -> (w1164:string[][])
                  }
                  frame True {
                    n677 = local read "Re-Calculated Values Cluster"() -> (w1172:T10)
                    n678 = Unbundle By Name(w1172) -> ("Trap Density-STS"=w1171:dbl)
                    n679 = Search 1D Array(1D array=w1174, element="Trap Density-VT (Traps/Vcm^2):") -> (index of element=w1181:i32)  [unwired: 1 in]
                    n680 = Divide(x=w1181, y=3) -> (x/y=w1182:dbl)
                    n681 = To Word Integer(number=w1182) -> (16bit integer=w1180:i16)
                    n682 = Format Value(format string="%#g", value (0)=w1171) -> (output string=w1185:string)  [unwired: 1 in]
                    n683 = Build Array(w1173, w1185) -> (w1178:string[])
                    n684 = Increment(x=w1180) -> (x+1=w1179:i16)
                    n685 = Insert Into Array(array=w1175, index (row)=w1179, new element=w1178) -> (w1176:string[][])  [unwired: 1 in]
                  }
                }
                n686 = local write "Save Array"(w1156) -> ()
              }
            }
            n687 = local read "New: Temp"() -> (w693:dbl)
            n688 = local read "New: Width"() -> (w694:dbl)
            n689 = local read "New: Length"() -> (w696:dbl)
            n690 = local read "Index"() -> (w695:string)
            n691 = To Single Precision Float(number=w693) -> (single precision float=w710:sgl)
            n692 = Number To Decimal String(number=w710) -> (decimal integer string=w705:string)  [unwired: 1 in]
            n693 = To Single Precision Float(number=w694) -> (single precision float=w709:sgl)
            n694 = To Single Precision Float(number=w696) -> (single precision float=w708:sgl)
            n695 = Strip Path(path=w692) -> (stripped path=w697:path)  [unwired: 1 out]
            n696 = Number To Decimal String(number=w708) -> (decimal integer string=w703:string)  [unwired: 1 in]
            n697 = Number To Decimal String(number=w709) -> (decimal integer string=w702:string)  [unwired: 1 in]
            n698 = Concatenate Strings("_", w705, "K") -> (w707:string)
            n699 = call "Build Text"("Temp"=w707, "Index"=w695, "Length"=w703, "Width"=w702) -> ("Result"=w701:string)  [unwired: 10 in, 1 out]
            n700 = Path To String(path=w697) -> (string=w699:string)
            n701 = Concatenate Strings(w699, "\\", w701) -> (w700:string)
            n702 = String To Path(string=w700) -> (path=w691:path)
          }
          frame #1 {
            n703 = flat-sequence {
              tunnel: w1189 -> [w1191]
              tunnel: w1188 -> [w1190]
              tunnel: [w1190] -> w1187
              tunnel: w1187 -> [w1197]
              tunnel: w1186 -> [w1196]
              frame #0 {
                n704 = Equal?(x=w1191, y=w1190) -> (x = y?=w1192:bool)
                n705 = case shown="False" w1192 {
                  tunnel: w1191 -> [w1195 _]
                  tunnel: w1190 -> [w1194 _]
                  frame False {
                    n706 = Move(source path=w1195, 9:TRUE, 10:w1194) -> ()  [unwired: 2 in, 3 out]
                  }
                  frame True {
                  }
                }
              }
              frame #1 {
                n707 = local write "Transfer File"(w1197) -> ()
                n708 = call-poly <vilib>:"Write To Spreadsheet File.vi"("2D data"=w1196, "file path (dialog if empty)"=w1197) -> ()  [unwired: 6 in, 1 out]
              }
            }
          }
        }
        n709 = Cluster To Array(cluster=w681) -> (array=w680:bool[])
        n710 = Boolean Array To Number(Boolean array=w680) -> (number=w679:u32)
        n711 = Equal To 0?(x=w679) -> (x = 0?=w678:bool)
        n712 = case shown="True" w678 {
          tunnel: [MegaAwesome_States."Read Data" w685] -> w677
          tunnel: w676 -> [_ w689]
          frame False {
          }
          frame True {
            n713 = Unbundle By Name(w689) -> ("Save Next"=w688:bool)
            n714 = Select(t=MegaAwesome_States."No Event", s=w688, f=MegaAwesome_States."Next File") -> (s? t:f=w685:T3)
          }
        }
      }
      frame "Exit" {
      }
      frame "Save Lines" {
      }
      frame "Export" {
        n715 = flat-sequence {
          frame #0 {
            n716 = stacked-sequence {
              frame #0 {
                n717 = local read "Independant Variable:"() -> (w1204:string)
                n718 = Equal?(x=w1204, y="Length (um):") -> (x = y?=w1205:bool)
                n719 = case shown="True" w1205 {
                  frame False {
                  }
                  frame True {
                    n720 = local write "X Axis Display Type"("1") -> ()
                    n721 = local write "Opj X Axis"("2") -> ()
                  }
                }
              }
              frame #1 {
                n722 = local read "Independant Variable:"() -> (w1209:string)
                n723 = Equal?(x=w1209, y="Sample Temp (K):") -> (x = y?=w1210:bool)
                n724 = case shown="True" w1210 {
                  frame False {
                  }
                  frame True {
                    n725 = local write "X Axis Display Type"("1") -> ()
                    n726 = local write "Opj X Axis"("1") -> ()
                  }
                }
              }
              frame #2 {
                n727 = local read "Independant Variable:"() -> (w1214:string)
                n728 = Equal?(x=w1214, y="Mobility-Sat (cm^2/Vs):") -> (x = y?=w1215:bool)
                n729 = case shown="True" w1215 {
                  frame False {
                  }
                  frame True {
                    n730 = local write "X Axis Display Type"("2") -> ()
                    n731 = local write "Opj X Axis"("2") -> ()
                  }
                }
              }
              frame #3 {
                n732 = local read "Independant Variable:"() -> (w1219:string)
                n733 = Equal?(x=w1219, y="Mobility-Lin (cm^2/Vs):") -> (x = y?=w1220:bool)
                n734 = case shown="True" w1220 {
                  frame False {
                  }
                  frame True {
                    n735 = local write "X Axis Display Type"("2") -> ()
                    n736 = local write "Opj X Axis"("2") -> ()
                  }
                }
              }
              frame #4 {
                n737 = local read "Independant Variable:"() -> (w1224:string)
                n738 = Equal?(x=w1224, y="On/Off I-Sat:") -> (x = y?=w1225:bool)
                n739 = case shown="True" w1225 {
                  frame False {
                  }
                  frame True {
                    n740 = local write "X Axis Display Type"("2") -> ()
                    n741 = local write "Opj X Axis"("2") -> ()
                  }
                }
              }
              frame #5 {
                n742 = local read "Independant Variable:"() -> (w1229:string)
                n743 = Equal?(x=w1229, y="Off I-Sat (A):") -> (x = y?=w1230:bool)
                n744 = case shown="True" w1230 {
                  frame False {
                  }
                  frame True {
                    n745 = local write "X Axis Display Type"("2") -> ()
                    n746 = local write "Opj X Axis"("2") -> ()
                  }
                }
              }
              frame #6 {
                n747 = local read "Independant Variable:"() -> (w1234:string)
                n748 = Equal?(x=w1234, y="Vt-Sat (V):") -> (x = y?=w1235:bool)
                n749 = case shown="True" w1235 {
                  frame False {
                  }
                  frame True {
                    n750 = local write "X Axis Display Type"("1") -> ()
                    n751 = local write "Opj X Axis"("1") -> ()
                  }
                }
              }
              frame #7 {
                n752 = local read "Independant Variable:"() -> (w1239:string)
                n753 = Equal?(x=w1239, y="STS-Sat (V/decade):") -> (x = y?=w1240:bool)
                n754 = case shown="True" w1240 {
                  frame False {
                  }
                  frame True {
                    n755 = local write "X Axis Display Type"("1") -> ()
                    n756 = local write "Opj X Axis"("1") -> ()
                  }
                }
              }
              frame #8 {
                n757 = local read "Independant Variable:"() -> (w1244:string)
                n758 = Equal?(x=w1244, y="Trap Density-VT (Traps/Vcm^2):") -> (x = y?=w1245:bool)
                n759 = case shown="True" w1245 {
                  frame False {
                  }
                  frame True {
                    n760 = local write "X Axis Display Type"("2") -> ()
                    n761 = local write "Opj X Axis"("2") -> ()
                  }
                }
              }
              frame #9 {
                n762 = local read "Independant Variable:"() -> (w1249:string)
                n763 = Equal?(x=w1249, y="Trap Density-STS (Traps/Vcm^2):") -> (x = y?=w1250:bool)
                n764 = case shown="True" w1250 {
                  frame False {
                  }
                  frame True {
                    n765 = local write "X Axis Display Type"("2") -> ()
                    n766 = local write "Opj X Axis"("2") -> ()
                  }
                }
              }
            }
          }
          frame #1 {
            n767 = local read "Transfer Folder"() -> (w1258:path)
            n768 = Build Path(base path=w1258, name or relative path="Stats") -> (appended path=w1259:path)
            n769 = local read "Origin Project File"() -> (w1270:path)
            n770 = call <vilib>:"Check if File or Folder Exists.vi"("path"=w1259) -> ("file or folder exists?"=w1274:bool, "dup path"=w1273:path)  [unwired: 8 in, 1 out]
            n771 = call <userlib>:"OA_ConnectToOrigin.vi"() -> ("error out"=w1271:errorcluster, "Origin.IOApplication"=w1272:refnum<k7>)  [unwired: 8 in]
            n772 = case shown="False" w1274 {
              tunnel: w1273 -> [w1447 w1448]
              tunnel: [w1446 w1448] -> w1257
              frame False {
                n773 = Create Folder(path (use dialog)=w1447) -> (created path=w1446:path)  [unwired: 2 in, 2 out]
              }
              frame True {
              }
            }
            n774 = call "File Dialog"("start path"=w1259) -> ("selected path"=w1261:path)  [unwired: 11 in, 3 out]
            n775 = call <userlib>:"OA_Load.vi"("error in (no error)"=w1271, "Path"=w1270, "Origin.IOApplication"=w1272) -> ("error out"=w1268:errorcluster, "Origin.IOApplication"=w1269:refnum<k7>)  [unwired: 1 out]
            n776 = call "OAExecute.vi"("script"="document -m 3;", "Error IO"=w1268, "Origin.IOApplication"=w1269) -> ("Error IO Out"=w1266:errorcluster, "Origin.IOApplication"=w1267:refnum<k7>)  [unwired: 1 in, 1 out]
            n777 = local read "Independant Variable:"() -> (w1254:string)
            n778 = stacked-sequence {
              tunnel: w1258 -> [w1285 w1315 w1327 w1349 w1369 w1390 w1411 w1434]
              tunnel: w1257 -> [w1286 w1314 w1328 w1348 w1370 w1391 w1412 w1435]
              tunnel: w1267 -> [w1288 w1312 w1330 w1351 w1372 w1393 w1414 w1437]
              tunnel: w1266 -> [w1287 w1313 w1329 w1350 w1371 w1392 w1413 w1436]
              tunnel: [_ _ _ _ _ _ _ w1432] -> w1256
              tunnel: [_ _ _ _ _ _ _ w1433] -> w1255
              tunnel: w1254 -> [w1284 w1305 w1326 w1347 w1368 w1389 w1410 w1431]
              frame #0 {
                n779 = local read "X Axis Display Type"() -> (w1276:string)
                n780 = local read "Opj X Axis"() -> (w1281:string)
                n781 = Concatenate Strings("window -a MOBLGraph;\nlayer.x.type=", w1281, "; layer.x.label.numFormat = ", w1276, "; Y3 = 1; X3 = 1;", "window -a MOBLTable;\nwindow -s TV;") -> (w1279:string)
                n782 = call "Param_Analysis_7_24b_JW.vi"("Independant Variable"=w1284, "error in (no error)"=w1287, "Data Folder"=w1285, "Parameter String"="Mobility-Lin (cm^2/Vs):", "Parameter Name"="Mobility-Lin", "Stats Folder"=w1286) -> ("error out"=w1290:errorcluster, "Output Array"=w1292:string[][], "Variables"=w1283:T27)  [unwired: 2 in, 1 out]
                n783 = call "Origin_Export_7_27a_JW.vi"("Input Conditions"=w1283, "Analysis Array"=w1292, "error in (no error)"=w1290, "Parameter Worksheet Name"="[MOBLTable]Mobilities", "Parameter Folder Script"="pe_cd \"Mobility-Lin\";", "Origin.IOApplication"=w1288) -> ("error out"=w1289:errorcluster, "reference out"=w1291:refnum<k7>)  [unwired: 3 in, 1 out]
                n784 = call "OAExecute.vi"("script"=w1279, "Error IO"=w1289, "Origin.IOApplication"=w1291) -> ()  [unwired: 1 in, 3 out]
              }
              frame #1 {
                n785 = local read "X Axis Display Type"() -> (w1297:string)
                n786 = local read "Opj X Axis"() -> (w1302:string)
                n787 = Concatenate Strings("window -a MOBSGraph;\nlayer.x.type=", w1302, "; layer.x.label.numFormat = ", w1297, "; Y3 = 1; X3 = 1;", "window -a MOBSTable;\nwindow -s TV;") -> (w1300:string)
                n788 = call "Param_Analysis_7_24b_JW.vi"("Independant Variable"=w1305, "error in (no error)"=w1313, "Data Folder"=w1315, "Parameter String"="Mobility-Sat (cm^2/Vs):", "Parameter Name"="Mobility-Sat", "Stats Folder"=w1314) -> ("error out"=w1308:errorcluster, "Output Array"=w1306:string[][], "Variables"=w1304:T27)  [unwired: 2 in, 1 out]
                n789 = call "Origin_Export_7_27a_JW.vi"("Input Conditions"=w1304, "Analysis Array"=w1306, "error in (no error)"=w1308, "Parameter Worksheet Name"="[MOBSTable]Mobilities", "Parameter Folder Script"="pe_cd \"Mobility-Sat\";", "Origin.IOApplication"=w1312) -> ("error out"=w1307:errorcluster, "reference out"=w1309:refnum<k7>)  [unwired: 3 in, 1 out]
                n790 = call "OAExecute.vi"("script"=w1300, "Error IO"=w1307, "Origin.IOApplication"=w1309) -> ()  [unwired: 1 in, 3 out]
              }
              frame #2 {
                n791 = local read "X Axis Display Type"() -> (w1318:string)
                n792 = local read "Opj X Axis"() -> (w1323:string)
                n793 = Concatenate Strings("window -a NSTSGraph;\nlayer.x.type=", w1323, "; layer.x.label.numFormat = ", w1318, "; Y3 = 1; X3 = 1;", "window -a NSTSTable;\nwindow -s TV;") -> (w1321:string)
                n794 = call "Param_Analysis_7_24b_JW.vi"("Independant Variable"=w1326, "error in (no error)"=w1329, "Data Folder"=w1327, "Parameter String"="Trap Density-STS (Traps/Vcm^2):", "Parameter Name"="Trap Density-STS", "Stats Folder"=w1328) -> ("error out"=w1333:errorcluster, "Output Array"=w1331:string[][], "Variables"=w1325:T27)  [unwired: 2 in, 1 out]
                n795 = call "Origin_Export_7_27a_JW.vi"("Input Conditions"=w1325, "Analysis Array"=w1331, "error in (no error)"=w1333, "Parameter Worksheet Name"="[NSTSTable]Trap Densities", "Parameter Folder Script"="pe_cd \"N-STS\";", "Origin.IOApplication"=w1330) -> ("error out"=w1332:errorcluster, "reference out"=w1334:refnum<k7>)  [unwired: 3 in, 1 out]
                n796 = call "OAExecute.vi"("script"=w1321, "Error IO"=w1332, "Origin.IOApplication"=w1334) -> ()  [unwired: 1 in, 3 out]
              }
              frame #3 {
                n797 = local read "X Axis Display Type"() -> (w1339:string)
                n798 = local read "Opj X Axis"() -> (w1344:string)
                n799 = call "Param_Analysis_7_24b_JW.vi"("Independant Variable"=w1347, "error in (no error)"=w1350, "Data Folder"=w1349, "Parameter String"="Trap Density-VT (Traps/Vcm^2):", "Parameter Name"="Trap Density-Vt", "Stats Folder"=w1348) -> ("error out"=w1354:errorcluster, "Output Array"=w1352:string[][], "Variables"=w1346:T27)  [unwired: 2 in, 1 out]
                n800 = Concatenate Strings("window -a NVtGraph;\nlayer.x.type=", w1344, "; layer.x.label.numFormat = ", w1339, "; Y3 = 1; X3 = 1;", "window -a NVtTable;\nwindow -s TV;") -> (w1342:string)
                n801 = call "Origin_Export_7_27a_JW.vi"("Input Conditions"=w1346, "Analysis Array"=w1352, "error in (no error)"=w1354, "Parameter Worksheet Name"="[NVTTable]Trap Densities", "Parameter Folder Script"="pe_cd \"N-Vt\";", "Origin.IOApplication"=w1351) -> ("error out"=w1353:errorcluster, "reference out"=w1355:refnum<k7>)  [unwired: 3 in, 1 out]
                n802 = call "OAExecute.vi"("script"=w1342, "Error IO"=w1353, "Origin.IOApplication"=w1355) -> ()  [unwired: 1 in, 3 out]
              }
              frame #4 {
                n803 = local read "X Axis Display Type"() -> (w1360:string)
                n804 = local read "Opj X Axis"() -> (w1365:string)
                n805 = Concatenate Strings("window -a OffIGraph;\nlayer.x.type=", w1365, "; layer.x.label.numFormat = ", w1360, "; Y3 = 1; X3 = 1;", "window -a OffITable;\nwindow -s TV;") -> (w1363:string)
                n806 = call "Param_Analysis_7_24b_JW.vi"("Independant Variable"=w1368, "error in (no error)"=w1371, "Data Folder"=w1369, "Parameter String"="Off I-Sat (A):", "Parameter Name"="Off I-Sat", "Stats Folder"=w1370) -> ("error out"=w1375:errorcluster, "Output Array"=w1373:string[][], "Variables"=w1367:T27)  [unwired: 2 in, 1 out]
                n807 = call "Origin_Export_7_27a_JW.vi"("Input Conditions"=w1367, "Analysis Array"=w1373, "error in (no error)"=w1375, "Parameter Worksheet Name"="[OffItable]OffCurrents", "Parameter Folder Script"="pe_cd \"OffI-Sat\";", "Origin.IOApplication"=w1372) -> ("error out"=w1374:errorcluster, "reference out"=w1376:refnum<k7>)  [unwired: 3 in, 1 out]
                n808 = call "OAExecute.vi"("script"=w1363, "Error IO"=w1374, "Origin.IOApplication"=w1376) -> ()  [unwired: 1 in, 3 out]
              }
              frame #5 {
                n809 = local read "X Axis Display Type"() -> (w1381:string)
                n810 = local read "Opj X Axis"() -> (w1386:string)
                n811 = Concatenate Strings("window -a OnOffGraph;\nlayer.x.type=", w1386, "; layer.x.label.numFormat = ", w1381, "; Y3 = 1; X3 = 1;", "window -a OnOffTable;\nwindow -s TV;") -> (w1384:string)
                n812 = call "Param_Analysis_7_24b_JW.vi"("Independant Variable"=w1389, "error in (no error)"=w1392, "Data Folder"=w1390, "Parameter String"="On/Off I-Sat:", "Parameter Name"="OnOff Ratio", "Stats Folder"=w1391) -> ("error out"=w1396:errorcluster, "Output Array"=w1394:string[][], "Variables"=w1388:T27)  [unwired: 2 in, 1 out]
                n813 = call "Origin_Export_7_27a_JW.vi"("Input Conditions"=w1388, "Analysis Array"=w1394, "error in (no error)"=w1396, "Parameter Worksheet Name"="[OnOffTable]On/Off Ratios", "Parameter Folder Script"="pe_cd \"OnOff-Ratio\";", "Origin.IOApplication"=w1393) -> ("error out"=w1395:errorcluster, "reference out"=w1397:refnum<k7>)  [unwired: 3 in, 1 out]
                n814 = call "OAExecute.vi"("script"=w1384, "Error IO"=w1395, "Origin.IOApplication"=w1397) -> ()  [unwired: 1 in, 3 out]
              }
              frame #6 {
                n815 = local read "X Axis Display Type"() -> (w1402:string)
                n816 = local read "Opj X Axis"() -> (w1407:string)
                n817 = call "Param_Analysis_7_24b_JW.vi"("Independant Variable"=w1410, "error in (no error)"=w1413, "Data Folder"=w1411, "Parameter String"="STS-Sat (V/decade):", "Parameter Name"="STS-Sat", "Stats Folder"=w1412) -> ("error out"=w1417:errorcluster, "Output Array"=w1415:string[][], "Variables"=w1409:T27)  [unwired: 2 in, 1 out]
                n818 = Concatenate Strings("window -a SGraph;\nlayer.x.type=", w1407, "; layer.x.label.numFormat = ", w1402, "; Y3 = 1; X3 = 1;", "window -a STable;\nwindow -s TV;") -> (w1405:string)
                n819 = call "Origin_Export_7_27a_JW.vi"("Input Conditions"=w1409, "Analysis Array"=w1415, "error in (no error)"=w1417, "Parameter Worksheet Name"="[STable]Threshold Swing", "Parameter Folder Script"="pe_cd \"STS-Sat\";", "Origin.IOApplication"=w1414) -> ("error out"=w1416:errorcluster, "reference out"=w1418:refnum<k7>)  [unwired: 3 in, 1 out]
                n820 = call "OAExecute.vi"("script"=w1405, "Error IO"=w1416, "Origin.IOApplication"=w1418) -> ()  [unwired: 1 in, 3 out]
              }
              frame #7 {
                n821 = local read "X Axis Display Type"() -> (w1423:string)
                n822 = local read "Opj X Axis"() -> (w1428:string)
                n823 = Concatenate Strings("window -a VtGraph;\nlayer.x.type=", w1428, "; layer.x.label.numFormat = ", w1423, "; Y3 = 1; X3 = 1;", "window -a VtTable;\nwindow -s TV;") -> (w1426:string)
                n824 = call "Param_Analysis_7_24b_JW.vi"("Independant Variable"=w1431, "error in (no error)"=w1436, "Data Folder"=w1434, "Parameter String"="Vt-Sat (V):", "Parameter Name"="Vt-Sat", "Stats Folder"=w1435) -> ("error out"=w1440:errorcluster, "Output Array"=w1438:string[][], "Variables"=w1430:T27)  [unwired: 2 in, 1 out]
                n825 = call "Origin_Export_7_27a_JW.vi"("Input Conditions"=w1430, "Analysis Array"=w1438, "error in (no error)"=w1440, "Parameter Worksheet Name"="[VtTable]Threshold Voltages", "Parameter Folder Script"="pe_cd \"Vt-Sat\";", "Origin.IOApplication"=w1437) -> ("error out"=w1439:errorcluster, "reference out"=w1441:refnum<k7>)  [unwired: 3 in, 1 out]
                n826 = call "OAExecute.vi"("script"=w1426, "Error IO"=w1439, "Origin.IOApplication"=w1441) -> ("Error IO Out"=w1432:errorcluster, "Origin.IOApplication"=w1433:refnum<k7>)  [unwired: 1 in, 1 out]
              }
            }
            n827 = Path To String(path=w1261) -> (string=w1260:string)
            n828 = call "OAExecute.vi"("script"="pe_cd /; ", "Error IO"=w1256, "Origin.IOApplication"=w1255) -> ("Error IO Out"=w1262:errorcluster, "Origin.IOApplication"=w1263:refnum<k7>)  [unwired: 1 in, 1 out]
            n829 = call <userlib>:"OASaveProject.vi"("path"=w1260, "Error IO"=w1262, "Origin.IOApplication"=w1263) -> ()  [unwired: 3 out]
          }
        }
      }
    }
    "Current State" <- w17
    "Folder Index" <- w10
    n830 = Select(t=50, s="Image Analysis?", f=10) -> (s? t:f=w4:i32)
    n831 = Wait (ms)(milliseconds to wait=w4) -> ()  [unwired: 1 out]
    n832 = Equal?(x=w19, y=MegaAwesome_States."Exit") -> (x = y?=w20:bool)
  }
